vi "Turbulence_3.2.vi"() -> ()   [LabVIEW 2018]
uses:
  <instrlib>/Mercury iXX/Public/Controls/Comms Transport Layer.ctl
  <userlib>/LightField Add-in and Automation SDK/Samples/LabVIEW Automation/lightfield-automation-labview/LightField Automation.lvclass
  C:/Program Files/Princeton Instruments/LightField/AddInViews/PrincetonInstruments.LightFieldViewV3.dll
  Program Files/Princeton Instruments/LightField/AddInViews/PrincetonInstruments.LightFieldViewV3.dll
  C:/Program Files/Princeton Instruments/LightField/PrincetonInstruments.LightFieldAddInSupportServices.dll
  Program Files/Princeton Instruments/LightField/PrincetonInstruments.LightFieldAddInSupportServices.dll
  <instrlib>/Keithley 2600 Series/Public/Channel.ctl
  <vilib>/DAQmx/read.llb/DAQmx Read (Counter DBL 1Chan 1Samp).vi
  <instrlib>/Mercury iXX/Public/Libraries/System/Open/Open System.vi
  <instrlib>/Mercury iXX/Public/Libraries/System/Read/Catalogue (Read).vi
  <vilib>/DAQmx/miscellaneous.llb/DAQmx Fill In Error Info.vi
  <instrlib>/Mercury iXX/Public/Libraries/Temperature/Open/Open Temperature Device.vi
  <instrlib>/Mercury iXX/Public/Libraries/Temperature/Signals/Read/Temperature (Read).vi
  <instrlib>/Quantum Composers 9000 Series 2.08/Quantum Composers 9000 Series.lvlib
  <instrlib>/Mercury iXX/Mercury iXX.lvlib
  <instrlib>/Mercury iXX/Public/Libraries/Temperature.lvlib
  <instrlib>/Keithley 2600 Series/Keithley 2600 Series.lvlib
  <instrlib>/Mercury iXX/Public/Libraries/System.lvlib
panel:
  out "Low Level\n(Ohms)":dbl format="%.1f"
  out "High Level\n(Ohms)":dbl format="%.1f"
  in  "Second Gate Width (us)":dbl=0.3
  in  "Initial Gate Width (us)":dbl=0.3
  in  "Second Gate Delay (us)":dbl=999.7
  in  "Initial Gate Delay (us)":dbl=1001.4
  in  "Extra Waits":i32
  in  "Error":bool
  in  "3He Check":bool=TRUE
  in  "File Exists":bool=TRUE
  out "Log":refnum<file>
  in  "Motor free":bool
  in  "RESTART":bool
  out "time string":string="12:58:38 PM"
  out "Timestamp":string
  out "Log Error":errorcluster
  in  "CLOSE":bool
  in  "RECORD":bool
  in  "Turbulence":T1(tab)
  out "Translation Error":bool caption="Error"
  in  "Camera Set":dbl=15.0 min=0.0 max=18.5 step=0.01 format="%.2f"
  in  "Mirror Set":dbl=10.0 min=0.0 max=25.4 step=0.01 format="%.2f"
  out "Camera":dbl=15.0 format="%.2f"
  out "Mirror":dbl=10.0 format="%.2f"
  in  "Home":bool
  in  "FROM FILE":bool
  in  "Script File":path
  in  "# Frames":i32=1000 min=0 step=1
  in  "New Background Movie":bool
  in  "On CCD Acc.":i32=3 min=0 step=1
  in  "Cycle time\n(ms)":i32=15 min=0 step=1
  in  "New Background Frame":bool
  out "Rate (Hz)":dbl
  out "Incident":dbl
  in  "BIN":u16(ring)=2 items=["1x1", "2x2", "4x4"]
  in  "MODE":u16(ring)=1 items=["Normal", "DIF"]
  in  "Enable":bool
  out "Rate (Hz)":dbl
  out "Detected":dbl
  in  "Script\nEnd":u32=1 step=1
  in  "Sample Space Pump":bool
  in  "Siphon Pump":bool
  in  "Neutron Shutter":bool
  in  "Manual Script Entry (0)":string
  in  "READY":bool=TRUE
  out "Power (mW)":dbl format="%_3f"
  out "Tank P2 (Torr)":string="0"
  in  "LIGHTFIELD":bool
  in  "SCRIPTING":bool
  in  "Top Coil":bool
  out "Tank P1 (Torr)":string="0.0"
  out "Cell (K)":dbl format="%.3f"
  out "Cryostat (K)":dbl format="%.3f"
  in  "Data Interval (s)":dbl=0.5 min=0.4 max=10.0 step=0.05
  in  "RUN/STOP":bool
  in  "Bottom Coil":bool
  in  "Bottom Coil (mA)":dbl min=-1000.0 max=1000.0 step=1e-05
  in  "Top Coil (mA)":dbl min=-1000.0 max=1000.0 step=1e-05
  in  "Percent Open":i32 min=0 max=100 step=5
  in  "COOLDOWN":bool
  in  "Script\n#":i32 step=1
  in  "Kill Switch":bool
  in  "DATA":bool
  out "Scripting Error":T2
  in  "Shutter Mode":u16(ring)=1 items=["Manual"=1, "XGate"=5]
  in  "REFILL":bool
  in  "AUTOFILL":bool
  in  "Low Level":dbl=10.0 format="%#_13g"
  out "L-He Level":dbl(slide) scale=0.0..100.0
  out "Liquid Level":dbl format="%_2f"
  out "Homing":bool
  in  "High Level":dbl=10.0 format="%#_13g"
  in  "Top":bool caption="Top Level"
  in  "Middle":bool
  in  "Bottom":bool
  in  "Fill":bool
  in  "Tare":bool
  out "Actual 3He\nTank Pressure":dbl min=0.0 max=100.0 step=5.0 format="%#.1g"
  out "Desired V2\nPressure (3He)":dbl min=0.0 max=100.0 step=5.0 format="%#.1f"
  in  "Desired Tank\nPressure (3He)":dbl min=0.0 max=100.0 step=0.01 format="%#.2f"
  in  "Log Pressure":bool
  out "4He Pressure (Torr)":string="-0.1"
  out "3He Pressure (Torr)":string="1"
  in  "Fill Time (s)":u32=10
  out "Overall Error":T3={"status"=TRUE, "codes"=-1073807343, "source"="VISA Open in Mercury iXX.lvlib:System.lvlib:Open System.vi->Turbulence_3.2.vi"}
  # "Camera Controls"
  # "Temperature Readout"
  # "Translation Controls"
  # "Neutron Counts"
  # "Automation"
  # "Pressure Readout"
  # "Relay Controls"
  # "Needle Valve Control"
  # "Heater Controls"
  # "Neutron Shutter"
  # "Optical Shutter"
  # "Siphon Pump"
  # "Laser Power Meter"
  # "Sample Space\nPump"
  # "V1 = 4075 mL"
  # "V2 = 15.5 mL"
  # "V3 = 78.8 mL"
  # "Quartz\nCell"
  # "4"
  # "3psi relief"
  # "MFC"
  # "V1"
  # "4L Tank"
  # "Turbo Pump"
  # "V2"
  # "V3"
  # "3"
  # "10psi relief"
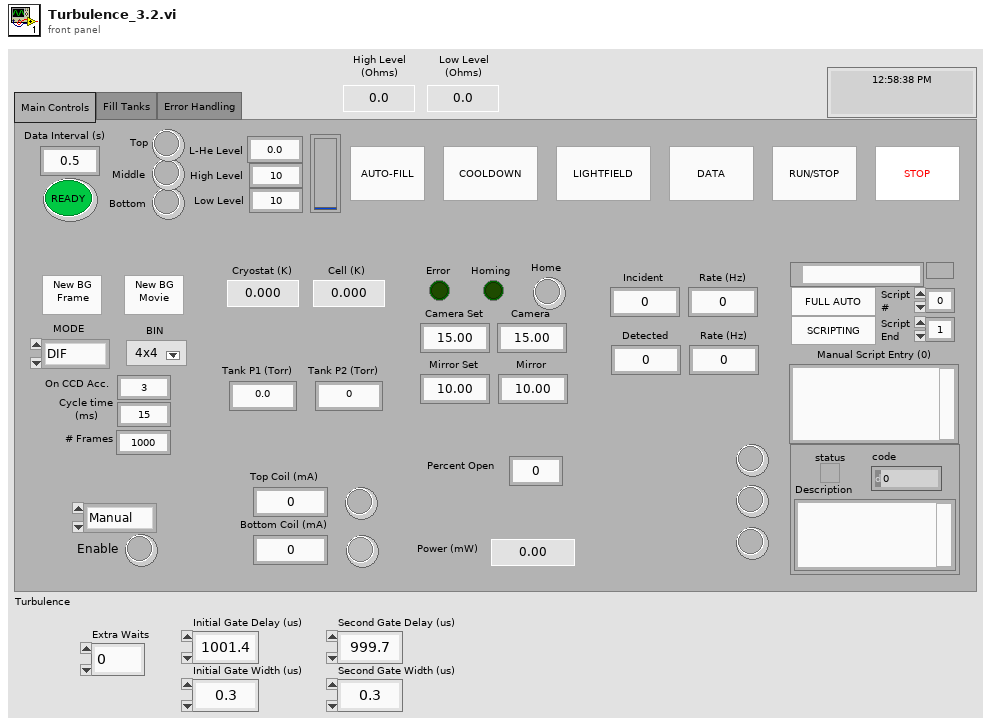
[diagram p1: front panel]
types:
  T1 = enum32{"Main Controls", "Fill Tanks", "Error Handling"}
  T2 = cluster{"status":bool, "code":i32, "Description":string}
  T3 = cluster{"status":bool, "codes":i32, "source":string}
  T4 = typedef "Mercury iXX.lvlib/Comms Transport Layer.ctl" = enum16{"Ethernet TCP/IP", "USB", "ISOBus - RS-232", "GPIB"}
  T5 = typedef "Mercury iXX.lvlib/Mercury Reference.ctl" = cluster{"Comms":refnum<visa-resource-name>, "Device ID":string[], "Comms Layer":T4, "Command":string, "Query reference":T6}
  T6 = typedef "Mercury iXX.lvlib/Query Dynamic Reference.ctl" = refnum<vi>
  T7 = enum32{"Current", "Voltage", "IV", "Resistance", "Power"}
  T8 = typedef "Keithley 2600 Series.lvlib/Channel.ctl" = enum32{"Channel A", "Channel B"}
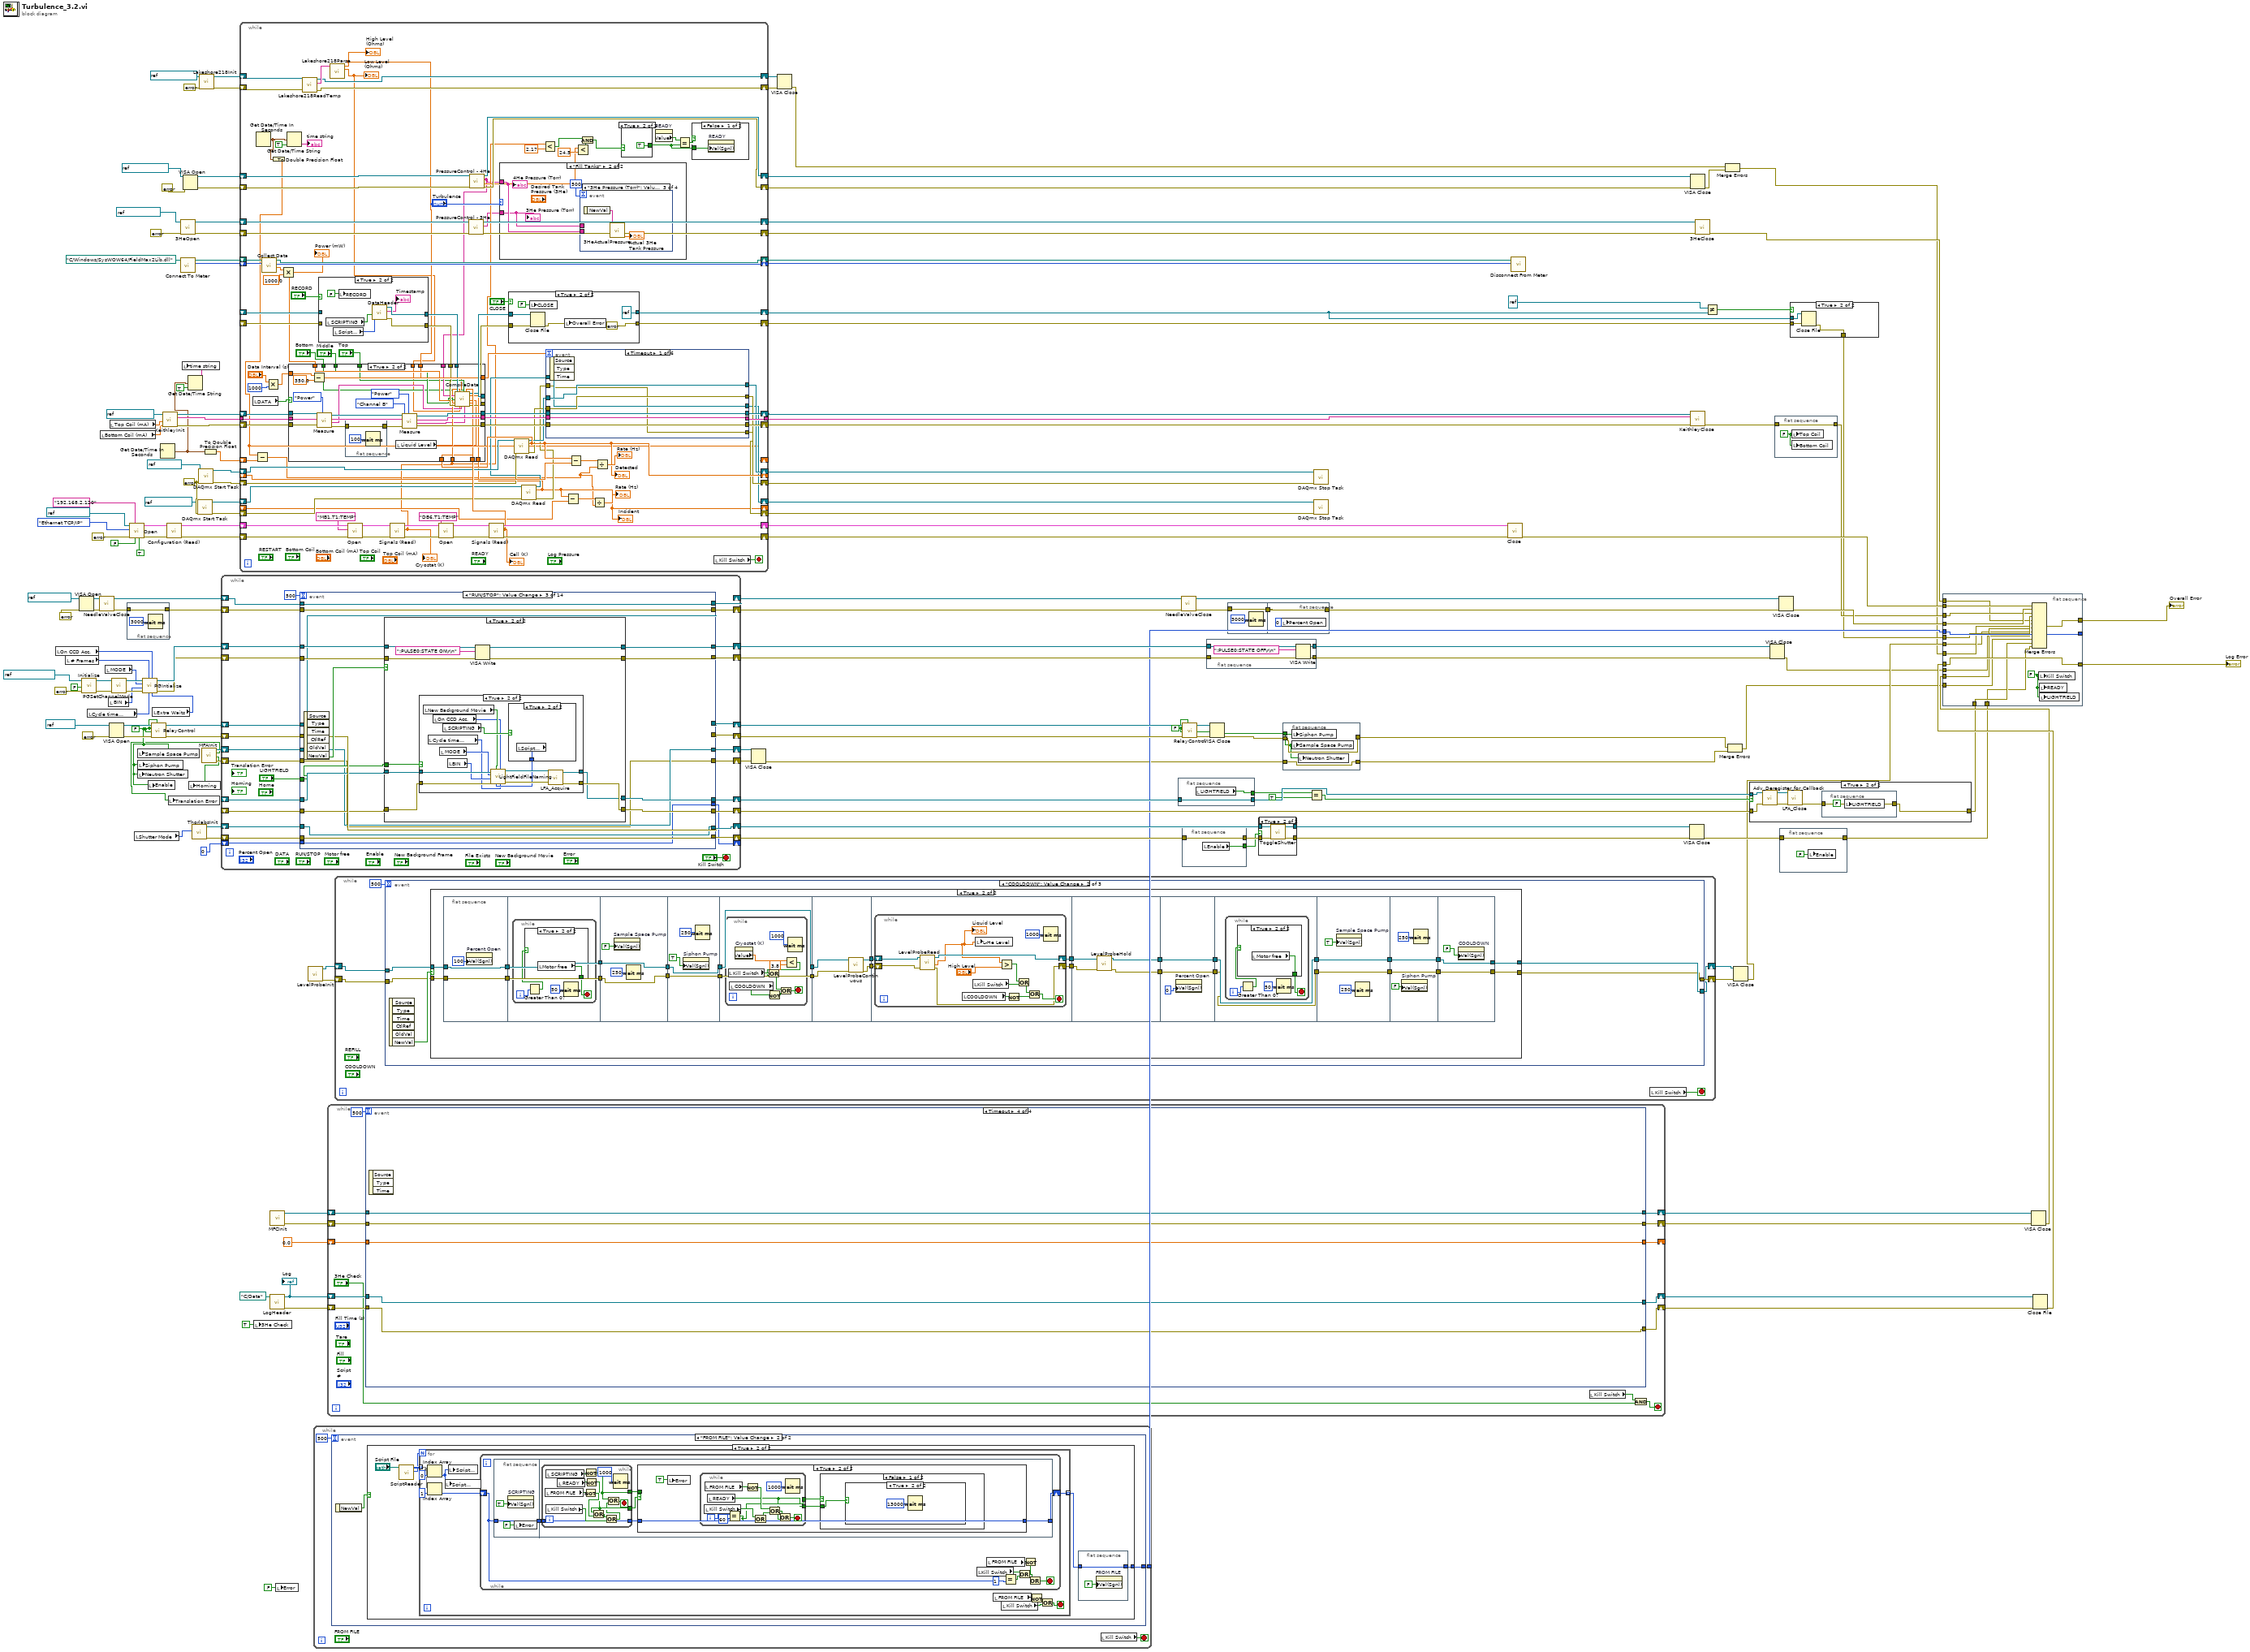
[diagram p0: block diagram]
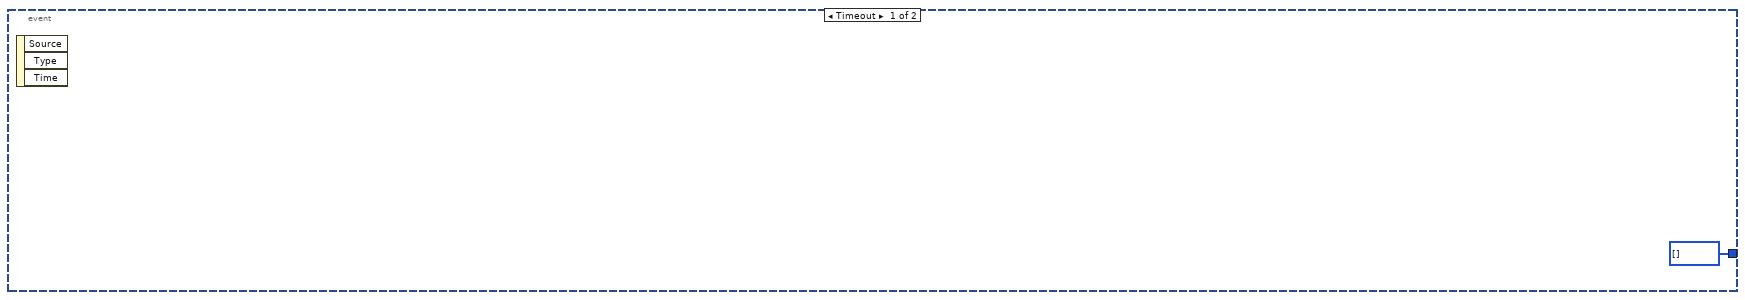
[diagram p2: hidden frame]
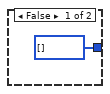
[diagram p3: hidden frame]
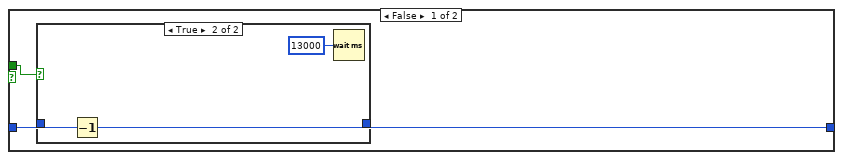
[diagram p4: hidden frame]
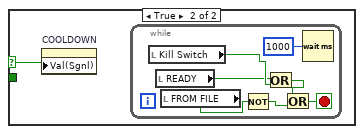
[diagram p7: hidden frame]
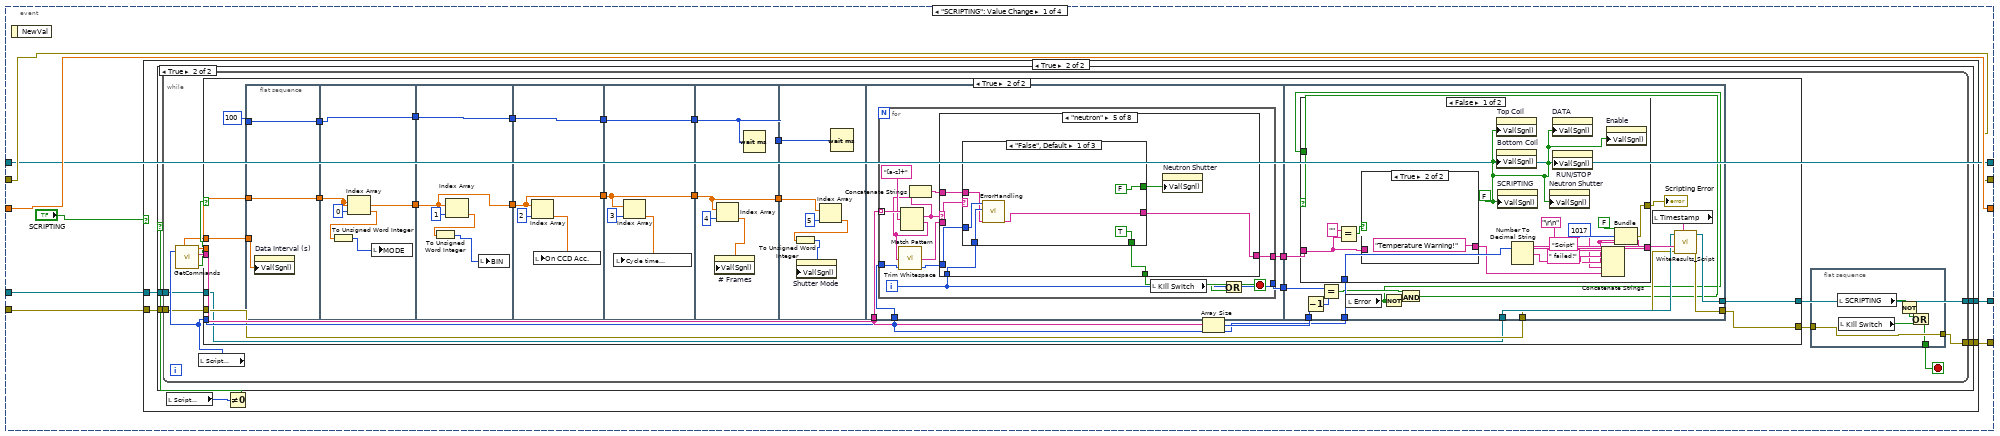
[diagram p10: hidden frame]
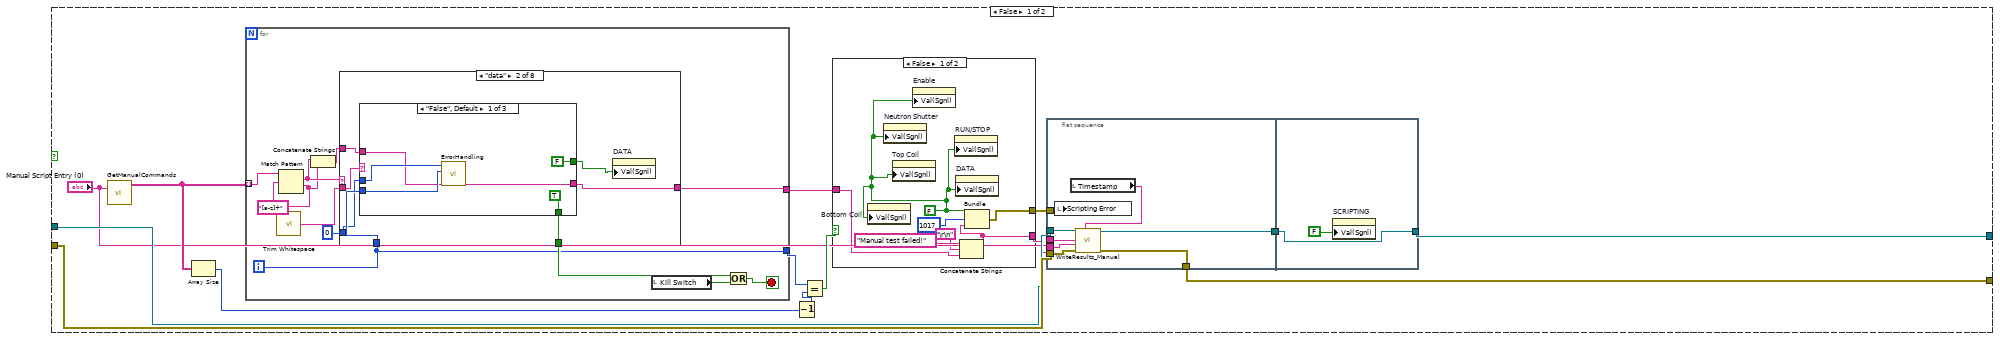
[diagram p12: hidden frame]
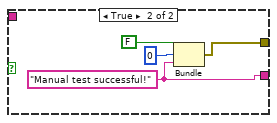
[diagram p13: hidden frame]
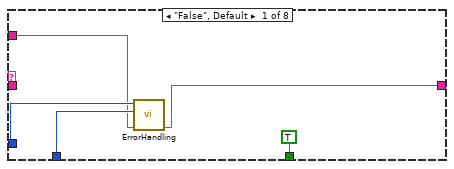
[diagram p14: hidden frame]
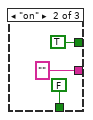
[diagram p15: hidden frame]
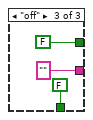
[diagram p16: hidden frame]
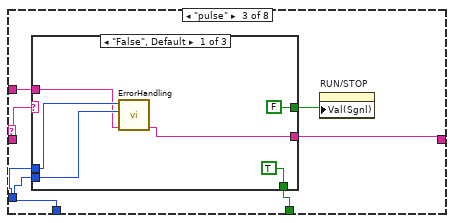
[diagram p17: hidden frame]
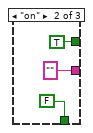
[diagram p18: hidden frame]
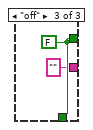
[diagram p19: hidden frame]
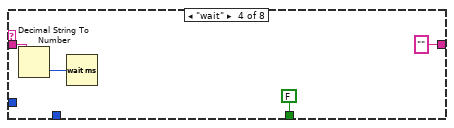
[diagram p20: hidden frame]
diagram:
  w65 = errorcluster {"status"=FALSE, "code"=0, "source"=""} ("error in")
  w101 = FALSE ("Siphon Pump")
  w87 = FALSE ("Siphon Pump")
  n1 = local read "On CCD Acc."() -> (w76:i32)
  n2 = local read "# Frames"() -> (w75:i32)
  n3 = VISA Open(error in (no error)=errorcluster {"status"=FALSE, "code"=0, "source"=""}, VISA resource name=refnum<visa-resource-name> "ZaberMotor") -> (VISA resource name=w82:refnum<visa-resource-name>, error out=w83:errorcluster)  [unwired: 3 in]
  n4 = call <instrlib>:"Initialize.vi"("error in (no error)"=errorcluster {"status"=FALSE, "code"=0, "source"=""}, "Reset? (T: Yes)"=FALSE, "VISA resource name"=refnum<visa-resource-name> "PulseGenerator" ("Pulse generater (COM3)")) -> ("error out"=w94:errorcluster, "VISA resource name out"=w92:refnum<visa-resource-name>)  [unwired: 7 in]
  n5 = local read "Cycle time\n(ms)"() -> (w44:i32)
  n6 = call "NeedleValveClose.vi"("error in (no error)"=w83, "VISA resource name"=w82) -> ("error out"=w84:errorcluster, "VISA resource name out"=w122:refnum<visa-resource-name>)  [unwired: 8 in]
  n7 = local read "Bottom Coil (mA)"() -> (w131:dbl)
  n8 = local read "MODE"() -> (w73:u16)
  n9 = local read "BIN"() -> (w74:u16)
  n10 = VISA Open(error in (no error)=errorcluster {"status"=FALSE, "code"=0, "source"=""} ("error in (no error) 2"), VISA resource name=refnum<visa-resource-name> "Relays" ("Pressure Gauge")) -> (VISA resource name=w143:refnum<visa-resource-name>, error out=w145:errorcluster)  [unwired: 3 in]
  n11 = local read "Top Coil (mA)"() -> (w132:dbl)
  n12 = call "PGSetChannelMode.vi"("error in"=w94, "VISA resource name"=w92) -> ("error out"=w93:errorcluster, "VISA resource name out"=w91:refnum<visa-resource-name>)  [unwired: 8 in]
  n13 = flat-sequence {
    tunnel: w84 -> [w170]
    tunnel: [w170] -> w123
    frame #0 {
      n14 = Wait (ms)(milliseconds to wait=u32 3000) -> ()  [unwired: 1 out]
    }
  }
  n15 = call-poly <instrlib>:"Open.vi"("Clear Previous Connections (False)"=TRUE, "ID Query (True)"=FALSE, "IP Address"="192.168.2.120", "error in (no error)"=errorcluster {"status"=FALSE, "code"=0, "source"=""}, "Comms Layer"=Comms_Transport_Layer."Ethernet TCP/IP", "VISA resource name"=refnum<visa-resource-name> "MercuryiTC") -> ("error out"=w163:errorcluster, "Mercury Reference Out"=w164:T5)  [unwired: 1 in, 3 out]
  n16 = local read "Shutter Mode"() -> (w77:u16)
  n17 = local write "Sample Space Pump"(w87) -> ()
  n18 = local write "Neutron Shutter"(w87) -> ()
  n19 = local write "Siphon Pump"(w87) -> ()
  n20 = local write "Enable"(w87) -> ()
  n21 = call "RelayControl.vi"("Neutron Shutter"=w87, "Error In"=w145, "Sample Space Pump"=w87, "Siphon Pump"=w87, "Relay In"=w143) -> ("Error Out"=w144:errorcluster, "Relay Out"=w142:refnum<visa-resource-name>)  [unwired: 5 in]
  n22 = local read "Extra Waits"() -> (w33:i32)
  n23 = call "PGIntialize.vi"("Extra Waits"=w33, "On CCD Accumulations"=w76, "Cycle time\n(ms)"=w44, "Number of Frames"=w75, "error in"=w93, "BIN"=w74, "MODE"=w73, "VISA resource name"=w91) -> ("error out"=w167:errorcluster, "VISA resource name out"=w168:refnum<visa-resource-name>)  [unwired: 2 in]
  n24 = Get Date/Time In Seconds() -> (seconds since 1Jan1904=w45:timestamp)
  n25 = call "KeithleyInit.vi"("Bottom Coil (mA)"=w131, "Top Coil (mA)"=w132, "KeithleyVISA In"=refnum<visa-resource-name> "Keithley2614B" ("VISA resource name")) -> ("error out"=w135:errorcluster, "Node Out"=w136:string, "KeithleyVISA Out"=w134:refnum<visa-resource-name>)  [unwired: 6 in]
  n26 = call-poly <instrlib>:"Configuration (Read).vi"("error in"=w163, "Mercury Reference In"=w164) -> ("error out"=w159:errorcluster, "Mercury Reference Out"=w160:T5)  [unwired: 6 in, 2 out]
  n27 = call "Connect To Meter.vi"("Location of FieldMax2Lib.dll in"=path "C:/Windows/SysWOW64/FieldMax2Lib.dll") -> ("Meter ID out"=w109:i32, "Location of FieldMax2Lib.dll out"=w108:path)  [unwired: 6 in, 1 out]
  n28 = call "3HeOpen.vi"("error in (no error)"=errorcluster {"status"=FALSE, "code"=0, "source"=""} ("error in (no error) 2"), "VISA resource name"=refnum<visa-resource-name> "3HePressure" ("Pressure Gauge")) -> ("error out"=w147:errorcluster, "VISA resource name out"=w146:refnum<visa-resource-name>)  [unwired: 8 in]
  n29 = VISA Open(error in (no error)=errorcluster {"status"=FALSE, "code"=0, "source"=""} ("error in (no error) 2"), VISA resource name=refnum<visa-resource-name> "TankPressure" ("Pressure Gauge")) -> (VISA resource name=w156:refnum<visa-resource-name>, error out=w157:errorcluster)  [unwired: 3 in]
  n30 = Get Date/Time String(seconds (now)=w45, want seconds? (F)=TRUE) -> (time string=w46:string)  [unwired: 1 in, 1 out]
  n31 = local write "time string"(w46) -> ()
  n32 = call "ThorlabsInit.vi"("Shutter Mode"=w77) -> ("error out"=w88:errorcluster, "VISA resource name out"=w89:refnum<visa-resource-name>)  [unwired: 9 in]
  n33 = call <vilib>:"DAQmx Start Task.vi"("task/channels in"=refnum<k21> "IncidentBeam", "error in"=w65) -> ("task out"=w67:refnum<k21>, "error out"=w66:errorcluster)  [unwired: 12 in]
  n34 = call <vilib>:"DAQmx Start Task.vi"("task/channels in"=refnum<k21> "Detector", "error in"=w65) -> ("task out"=w70:refnum<k21>, "error out"=w69:errorcluster)  [unwired: 12 in]
  n35 = call "Lakeshore218Init.vi"("error in (no error)"=errorcluster {"status"=FALSE, "code"=0, "source"=""}, "VISA resource name"=refnum<visa-resource-name> "Lakeshore218") -> ("error out"=w14:errorcluster, "VISA resource name out"=w15:refnum<visa-resource-name>)  [unwired: 8 in]
  n36 = call "MFAInit.vi"() -> ("error out"=w31:errorcluster, "Homing"=w25:bool, "Timeout"=w24:bool, "reference out"=w32:refnum<visa-resource-name>)  [unwired: 8 in]
  n37 = local write "Translation Error"(w24) -> ()
  n38 = local write "Homing"(w25) -> ()
  n39 = To Double Precision Float(number=w45) -> (double precision float=w48:dbl)
  n40 = while {
    shift-right: [w199] -> w55
    shift-left: _ -> [w197]
    shift-right: [w200] -> w61
    shift-left: _ -> [w198]
    shift-right: [w193] -> w116
    shift-left: w168 -> [w195]
    shift-right: [w194] -> w117
    shift-left: w167 -> [w196]
    shift-right: [w189] -> w121
    shift-left: w144 -> [w192]
    shift-right: [w190] -> w119
    shift-left: w142 -> [w191]
    shift-right: [w184] -> w148
    shift-left: w123 -> [w187]
    shift-right: [w185] -> w149
    shift-left: w122 -> [w186]
    shift-right: [w181] -> w57
    shift-left: w89 -> [w178]
    shift-right: [w180] -> w51
    shift-left: w88 -> [w179]
    shift-right: [w175] -> w30
    shift-left: w32 -> [w177]
    shift-right: [w174] -> w29
    shift-left: w31 -> [w176]
    shift-right: [w172] -> _
    shift-left: 0 -> [w173]
    stop <- "Kill Switch" stop-if-true
    n41 = event shown="[2] \"RUN/STOP\": Value Change" {
      selector: _ -> [_ _ _ _ _ _ _ _ _ _ _ _ _ _]
      dyn-events: _ -> [_ _ _ _ _ _ _ _ _ _ _ _ _ _]
      timeout: 500 -> [_ _ _ _ _ _ _ _ _ _ _ _ _ _]
      tunnel: w196 -> [w227 w252 w336 w385 w406 w458 w526 w548 w566 w592 w620 w677 w700 w735]
      tunnel: w195 -> [w226 w251 w337 w386 w405 w459 w527 w547 w565 w591 w621 w678 w701 w736]
      tunnel: w198 -> [w228 w255 w327 w377 w408 w462 w524 w551 w570 w583 w616 w673 w691 w733]
      tunnel: w197 -> [w229 w256 w328 w378 w409 w463 w525 w552 w569 w584 w617 w674 w692 w734]
      tunnel: [w228 w257 w326 w377 w408 w450 w524 w551 w570 w583 w616 w673 w691 w726] -> w200
      tunnel: [w229 w258 w325 w378 w409 w442 w525 w552 w569 w584 w617 w674 w692 w725] -> w199
      tunnel: [w227 w252 w339 w385 w406 w448 w526 w548 w566 w589 w620 w677 w700 w735] -> w194
      tunnel: [w226 w251 w338 w386 w405 w455 w527 w547 w565 w590 w621 w678 w701 w736] -> w193
      tunnel: w192 -> [w224 w253 w333 w383 w411 w457 w533 w550 w568 w585 w618 w675 w698 w728]
      tunnel: w191 -> [w225 w254 w334 w384 w410 w456 w532 w549 w567 w586 w619 w676 w699 w727]
      tunnel: [w225 w254 w334 w384 w410 w456 w529 w549 w567 w586 w619 w676 w699 w727] -> w190
      tunnel: [w224 w253 w333 w383 w411 w457 w528 w550 w568 w585 w618 w675 w698 w728] -> w189
      tunnel: w187 -> [w223 w250 w332 w387 w394 w461 w523 w546 w564 w587 w622 w679 w702 w737]
      tunnel: w186 -> [w222 w249 w331 w388 w407 w460 w522 w545 w563 w588 w623 w680 w703 w738]
      tunnel: [w222 w249 w331 w388 w404 w460 w522 w545 w563 w588 w623 w680 w703 w738] -> w185
      tunnel: [w223 w250 w332 w387 w396 w461 w523 w546 w564 w587 w622 w679 w702 w737] -> w184
      tunnel: "LIGHTFIELD" -> [_ _ w324 w382 _ w444 _ _ _ w579 _ _ _ w724]
      tunnel: w178 -> [w220 w247 w330 w380 w402 w454 w520 w544 w574 w582 w615 w672 w690 w732]
      tunnel: w179 -> [w221 w246 w329 w379 w401 w453 w519 w543 w573 w581 w614 w671 w689 w731]
      tunnel: [w220 w247 w330 w380 w402 w454 w520 w541 w571 w582 w615 w672 w690 w732] -> w181
      tunnel: [w221 w246 w329 w379 w401 w453 w519 w542 w572 w581 w614 w671 w689 w731] -> w180
      tunnel: w177 -> [w210 w245 w323 w376 w393 w439 w516 w537 w561 w577 w613 w667 w694 w729]
      tunnel: w176 -> [w211 w244 w322 w375 w392 w438 w515 w536 w560 w576 w612 w666 w693 w730]
      tunnel: [w212 w245 w323 w376 w393 w439 w516 w537 w561 w577 w613 w665 w688 w729] -> w175
      tunnel: [w207 w244 w322 w375 w392 w438 w515 w536 w560 w576 w612 w664 w687 w730] -> w174
      tunnel: w173 -> [w202 w243 w321 w374 w391 w437 w514 w535 w559 w575 w611 w659 w685 w723]
      tunnel: [w201 w243 w321 w374 w391 w437 w514 w535 w559 w575 w611 w659 w685 w723] -> w172
      event Timeout {
        n42 = event-data() -> ()  [unwired: 1 in, 3 out]
        n43 = call <instrlib>:"tell current position.vi"("error in"=w211, "Axis in"=1, "VISA Handle in"=w210) -> ("error out"=w208:errorcluster, "Current position (units)"=w204:dbl, "VISA Handle out"=w218:refnum<visa-resource-name>, "TimeoutFlag"=w216:bool)  [unwired: 2 in, 1 out]
        "Camera" <- w204
        n44 = flat-sequence {
          tunnel: w208 -> [w242]
          tunnel: [w242] -> w213
          frame #0 {
            n45 = Wait (ms)(milliseconds to wait=u32 50) -> ()  [unwired: 1 out]
          }
        }
        n46 = call <instrlib>:"tell current position.vi"("error in"=w213, "Axis in"=2, "VISA Handle in"=w218) -> ("error out"=w207:errorcluster, "Current position (units)"=w203:dbl, "VISA Handle out"=w212:refnum<visa-resource-name>, "TimeoutFlag"=w215:bool)  [unwired: 2 in, 1 out]
        "Mirror" <- w203
        n47 = Or(x=w216, y=w215) -> (x .or. y?=w214:bool)
        n48 = local write "Translation Error"(w214) -> ()
        n49 = local read "Homing"() -> (w209:bool)
        n50 = Equal?(x=w202, y=0) -> (x = y?=w206:bool)
        n51 = case shown="True" w209 {
          tunnel: w203 -> [_ w235]
          tunnel: w204 -> [_ w234]
          frame False {
          }
          frame True {
            w236 = 0.0 ("y")
            n52 = Equal?(x=w235, y=w236) -> (x = y?=w239:bool)
            n53 = Equal?(x=w234, y=w236) -> (x = y?=w238:bool)
            n54 = And(x=w239, y=w238) -> (x .and. y?=w237:bool)
            n55 = case shown="False" w237 {
              frame False {
              }
              frame True {
                n56 = local write "Homing"(FALSE ("Homing")) -> ()
              }
            }
          }
        }
        n57 = case shown="True" w206 {
          tunnel: w204 -> [_ w232]
          tunnel: w203 -> [_ w231]
          tunnel: w202 -> [w230 _]
          tunnel: [w230 1] -> w201
          frame False {
          }
          frame True {
            n58 = local write "Camera Set"(w232) -> ()
            n59 = local write "Mirror Set"(w231) -> ()
          }
        }
      }
      event "LIGHTFIELD": Value Change {
        n60 = event-data() -> ("NewVal"=w248:bool)  [unwired: 1 in, 5 out]
        n61 = case shown="False" w248 {
          tunnel: [refnum<class "LightField Automation.lvclass"> refnum ("LightField Automation out") w274] -> w258
          tunnel: [errorcluster {"status"=FALSE, "code"=0, "source"=""} ("error out") w273] -> w257
          tunnel: w256 -> [w263 _]
          tunnel: w255 -> [w262 _]
          frame False {
            n62 = call <userlib>:"Adv_Deregister_for_Callback.vi"("error in (no error)"=w262, "LightField Automation in"=w263) -> ("error out"=w264:errorcluster, "LightField Automation out"=w265:refnum<class "LightField Automation.lvclass">)  [unwired: 8 in]
            n63 = call <userlib>:"LFA_Close.vi"("error in (no error)"=w264, "LightField Automation in"=w265) -> ("error out"=w259:errorcluster)  [unwired: 8 in, 1 out]
            n64 = local write "Overall Error"(w259) -> ()
          }
          frame True {
            n65 = call <userlib>:"LFA_Initialize.vi"("error in (no error)"=errorcluster {"status"=FALSE, "code"=0, "source"=""}) -> ("error out"=w283:errorcluster, "LightField Automation out"=w282:refnum<class "LightField Automation.lvclass">)  [unwired: 9 in]
            n66 = call <userlib>:"Adv_Register_for_Callback.vi"("error in (no error)"=w283, "LightField Automation in"=w282) -> ("error out"=w281:errorcluster, "LightField Automation out"=w280:refnum<class "LightField Automation.lvclass">)  [unwired: 8 in]
            n67 = call <userlib>:"Exp_SetExperiment.vi"("error in (no error)"=w281, "ExperimentName"="20190801_DIF", "LightField Automation in"=w280) -> ("error out"=w267:errorcluster, "LightField Automation out"=w266:refnum<class "LightField Automation.lvclass">)  [unwired: 7 in]
            n68 = flat-sequence {
              tunnel: [w291] -> w271
              tunnel: [w290] -> w270
              tunnel: [w289] -> w269
              tunnel: [w292] -> w268
              tunnel: w267 -> [w295]
              tunnel: w266 -> [w293]
              tunnel: [w306] -> w277
              tunnel: [w305] -> w276
              tunnel: [w304] -> w275
              tunnel: [w303] -> w272
              tunnel: w271 -> [w303]
              tunnel: w270 -> [w306]
              tunnel: w269 -> [w305]
              tunnel: w268 -> [w304]
              tunnel: w277 -> [w311]
              tunnel: w276 -> [w312]
              tunnel: w275 -> [w310]
              tunnel: [w309] -> w274
              tunnel: [w308] -> w273
              tunnel: w272 -> [w307]
              frame #0 {
                n69 = local read "On CCD Acc."() -> (w301:i32)
                n70 = local read "Cycle time\n(ms)"() -> (w288:i32)
                n71 = local read "# Frames"() -> (w299:i32)
                n72 = local read "Second Gate Width (us)"() -> (w285:dbl)
                n73 = local read "BIN"() -> (w300:u16)
                n74 = local read "Second Gate Delay (us)"() -> (w284:dbl)
                n75 = local read "Initial Gate Width (us)"() -> (w286:dbl)
                n76 = call <userlib>:"Exp_ICCD_SetIntensifierGain.vi"("error in (no error)"=w295, "Intensifier Gain"=100, "LightField Automation in"=w293) -> ("error out"=w297:errorcluster, "LightField Automation out"=w296:refnum<class "LightField Automation.lvclass">)  [unwired: 7 in]
                n77 = local read "Initial Gate Delay (us)"() -> (w287:dbl)
                n78 = local read "MODE"() -> (w302:u16)
                n79 = local read "Log"() -> (w298:refnum<file>)
                n80 = call "LightFieldInit.vi"("LightField Automation in"=w296, "MODE"=w302, "BIN"=w300, "error in"=w297, "Initial Gate Delay (us)"=w287, "Initial Gate Width (us)"=w286, "Number of Frames"=w299, "File Path"=w298, "On CCD Accumulations"=w301, "Second Gate Delay (us)"=w284, "Second Gate Width (us)"=w285) -> ("LightField Automation out"=w289:refnum<class "LightField Automation.lvclass">, "error out"=w290:errorcluster)  [unwired: 7 in]
                n81 = call "LightFieldBackgroundNaming.vi"("Cycle time\n(ms)"=w288, "On CCD Acc."=w301, "BIN"=w300, "MODE"=w302) -> ("FilePath"=w292:string, "Exists"=w291:bool)  [unwired: 5 in, 1 out]
              }
              frame #1 {
                n82 = local write "File Exists"(w303) -> ()
              }
              frame #2 {
                n83 = case shown="False" w307 {
                  tunnel: w312 -> [w315 w320]
                  tunnel: w311 -> [w314 w319]
                  tunnel: w310 -> [_ w318]
                  tunnel: [w315 w317] -> w309
                  tunnel: [w314 w316] -> w308
                  frame False {
                    n84 = property on="New Background Frame" class="Bool (strict)"("Val(Sgnl)"=TRUE ("Value (Signaling)")) -> ()  [unwired: 2 in, 2 out]
                  }
                  frame True {
                    n85 = call "LightFieldChangeBackground.vi"("error in"=w319, "FilePath"=w318, "LightField Automation in"=w320) -> ("error out"=w316:errorcluster, "LightField Automation out"=w317:refnum<class "LightField Automation.lvclass">)  [unwired: 7 in]
                  }
                }
              }
            }
          }
        }
      }
      event "RUN/STOP": Value Change {
        n86 = event-data() -> ("NewVal"=w335:bool)  [unwired: 1 in, 5 out]
        n87 = case shown="True" w335 {
          tunnel: [w343 w356] -> w339
          tunnel: [w344 w355] -> w338
          tunnel: w337 -> [w345 w354]
          tunnel: w336 -> [w346 w353]
          tunnel: w328 -> [w341 w351]
          tunnel: w327 -> [w340 w350]
          tunnel: [w340 w349] -> w326
          tunnel: [w341 w348] -> w325
          tunnel: w324 -> [_ w347]
          frame False {
            n88 = VISA Write(VISA resource name=w345, write buffer=":PULSE0:STATE OFF\r\n" ("format string"), error in (no error)=w346) -> (VISA resource name out=w344:refnum<visa-resource-name>, error out=w343:errorcluster)  [unwired: 1 out]
          }
          frame True {
            n89 = case shown="True" w347 {
              tunnel: w350 -> [w357 w369]
              tunnel: w351 -> [w358 w367]
              tunnel: [w358 w371] -> w348
              tunnel: [w357 w370] -> w349
              frame False {
              }
              frame True {
                n90 = local read "New Background Movie"() -> (w361:bool)
                n91 = local read "Cycle time\n(ms)"() -> (w359:i32)
                n92 = local read "On CCD Acc."() -> (w360:i32)
                n93 = local read "MODE"() -> (w364:u16)
                n94 = local read "SCRIPTING"() -> (w362:bool)
                n95 = local read "BIN"() -> (w365:u16)
                n96 = case shown="True" w362 {
                  tunnel: [-1 ("Script\n#") w373] -> w363
                  frame False {
                  }
                  frame True {
                    n97 = local read "Script\n#"() -> (w373:i32)
                  }
                }
                n98 = call "LightFieldFileNaming.vi"("Cycle time\n(ms)"=w359, "On CCD Acc."=w360, "Script#"=w363, "BG"=w361, "error in"=w369, "BIN"=w365, "MODE"=w364, "LightField Automation in"=w367) -> ("error out"=w368:errorcluster, "LightField Automation out"=w366:refnum<class "LightField Automation.lvclass">)  [unwired: 2 in]
                n99 = call <instrlib>:"LFA_Acquire.vi"("error in (no error)"=w368, "LightField Automation in"=w366) -> ("error out"=w370:errorcluster, "LightField Automation out"=w371:refnum<class "LightField Automation.lvclass">)  [unwired: 8 in]
              }
            }
            n100 = VISA Write(VISA resource name=w354, write buffer=":PULSE0:STATE ON\r\n" ("format string"), error in (no error)=w353) -> (VISA resource name out=w355:refnum<visa-resource-name>, error out=w356:errorcluster)  [unwired: 1 out]
          }
        }
      }
      event "DATA": Value Change {
        n101 = event-data() -> ("NewVal"=w381:bool)  [unwired: 1 in, 5 out]
        n102 = case shown="False" w381 {
          tunnel: w382 -> [_ _]
          frame False {
            n103 = local write "CLOSE"(TRUE ("CLOSE")) -> ()
          }
          frame True {
            n104 = local write "RECORD"(TRUE ("RECORD")) -> ()
          }
        }
      }
      event "Percent Open": Value Change {
        n105 = event-data() -> ("OldVal"=w403:i32, "NewVal"=w412:i32)  [unwired: 1 in, 4 out]
        n106 = flat-sequence {
          tunnel: w394 -> [w414]
          tunnel: [w414] -> w395
          frame #0 {
            n107 = property on="Motor free" class="Bool (strict)"("Val(Sgnl)"=FALSE ("Value (Signaling)")) -> ()  [unwired: 2 in, 2 out]
          }
        }
        n108 = Subtract(x=w412, y=w403) -> (x-y=w398:i32)
        n109 = Greater Than 0?(x=w398) -> (x > 0?=w399:bool)
        n110 = Equal To 0?(x=w412) -> (x = 0?=w400:bool)
        n111 = case shown="False" w400 {
          tunnel: w407 -> [w420 w436]
          tunnel: w395 -> [w421 w435]
          tunnel: [w419 w434] -> w404
          tunnel: [w418 w433] -> w397
          tunnel: w399 -> [w422 _]
          tunnel: w398 -> [w417 _]
          frame False {
            n112 = case shown="True" w422 {
              tunnel: w421 -> [w426 w432]
              tunnel: w420 -> [w427 w431]
              tunnel: [w425 w430] -> w419
              tunnel: [w424 w429] -> w418
              tunnel: w417 -> [w423 w428]
              frame False {
                n113 = call "NeedleValveClose - Encoder.vi"("error in (no error)"=w426, "Percent Difference"=w423, "VISA resource name"=w427) -> ("error out"=w424:errorcluster, "VISA resource name out"=w425:refnum<visa-resource-name>)  [unwired: 7 in]
              }
              frame True {
                n114 = call "NeedleValveOpen - Encoder.vi"("error in (no error)"=w432, "Percent Difference"=w428, "VISA resource name"=w431) -> ("error out"=w429:errorcluster, "VISA resource name out"=w430:refnum<visa-resource-name>)  [unwired: 7 in]
              }
            }
          }
          frame True {
            n115 = call "NeedleValveClose.vi"("error in (no error)"=w435, "VISA resource name"=w436) -> ("error out"=w433:errorcluster, "VISA resource name out"=w434:refnum<visa-resource-name>)  [unwired: 8 in]
          }
        }
        n116 = flat-sequence {
          tunnel: w397 -> [w416]
          tunnel: [w416] -> w396
          frame #0 {
            n117 = property on="Motor free" class="Bool (strict)"("Val(Sgnl)"=TRUE ("Value (Signaling)")) -> ()  [unwired: 2 in, 2 out]
          }
        }
      }
      event "Cycle time\n(ms)", "# Frames", "MODE", "BIN", "On CCD Acc.", "Extra Waits": Value Change {
        n118 = event-data() -> ()  [unwired: 1 in, 1 out]
        n119 = case shown="True" w444 {
          tunnel: w463 -> [w504 w512]
          tunnel: w462 -> [w505 w513]
          tunnel: [w504 w511] -> w443
          tunnel: [w505 w510] -> w451
          tunnel: "On CCD Acc." -> [_ w508]
          tunnel: "# Frames" -> [_ w509]
          tunnel: "BIN" -> [_ w507]
          tunnel: "MODE" -> [_ w506]
          frame False {
          }
          frame True {
            n120 = call "LightFieldParams.vi"("On CCD Accumulations"=w508, "Number of Frames"=w509, "error in"=w513, "BIN"=w507, "MODE"=w506, "LightField Automation in"=w512) -> ("error out"=w510:errorcluster, "LightField Automation out"=w511:refnum<class "LightField Automation.lvclass">)  [unwired: 4 in]
          }
        }
        n121 = call "PGIntialize.vi"("Extra Waits"="Extra Waits", "On CCD Accumulations"="On CCD Acc.", "Cycle time\n(ms)"="Cycle time\n(ms)", "Number of Frames"="# Frames", "error in"=w458, "BIN"="BIN", "MODE"="MODE", "VISA resource name"=w459) -> ("error out"=w449:errorcluster, "VISA resource name out"=w455:refnum<visa-resource-name>)  [unwired: 2 in]
        n122 = case shown="True" w444 {
          tunnel: w451 -> [w466 w476]
          tunnel: [w466 w475] -> w450
          tunnel: w449 -> [w465 w474]
          tunnel: [w465 w473] -> w448
          tunnel: "On CCD Acc." -> [_ w472]
          tunnel: "BIN" -> [_ w471]
          tunnel: "MODE" -> [_ w470]
          tunnel: w443 -> [w464 w469]
          tunnel: [w464 w468] -> w442
          tunnel: "Cycle time\n(ms)" -> [_ w467]
          frame False {
          }
          frame True {
            n123 = flat-sequence {
              tunnel: w476 -> [w480]
              tunnel: [w479] -> w475
              tunnel: w474 -> [w488]
              tunnel: [w488] -> w473
              tunnel: w472 -> [w487]
              tunnel: w471 -> [w486]
              tunnel: w470 -> [w485]
              tunnel: w469 -> [w481]
              tunnel: [w478] -> w468
              tunnel: w467 -> [w477]
              frame #0 {
                n124 = call "LightFieldBackgroundNaming.vi"("Cycle time\n(ms)"=w477, "On CCD Acc."=w487, "BIN"=w486, "MODE"=w485) -> ("FilePath"=w482:string, "Exists"=w484:bool)  [unwired: 5 in, 1 out]
                n125 = flat-sequence {
                  tunnel: w484 -> [w489]
                  tunnel: [w489] -> w483
                  tunnel: w483 -> [w495]
                  tunnel: w482 -> [w494]
                  tunnel: w481 -> [w493]
                  tunnel: w480 -> [w492]
                  tunnel: [w491] -> w479
                  tunnel: [w490] -> w478
                  frame #0 {
                    n126 = local write "File Exists"(w489) -> ()
                  }
                  frame #1 {
                    n127 = case shown="True" w495 {
                      tunnel: w494 -> [_ w503]
                      tunnel: w493 -> [w497 w502]
                      tunnel: w492 -> [w496 w501]
                      tunnel: [w496 w500] -> w491
                      tunnel: [w497 w499] -> w490
                      frame False {
                        n128 = property on="New Background Frame" class="Bool (strict)"("Val(Sgnl)"=TRUE ("Value (Signaling)")) -> ()  [unwired: 2 in, 2 out]
                      }
                      frame True {
                        n129 = call "LightFieldChangeBackground.vi"("error in"=w501, "FilePath"=w503, "LightField Automation in"=w502) -> ("error out"=w500:errorcluster, "LightField Automation out"=w499:refnum<class "LightField Automation.lvclass">)  [unwired: 7 in]
                      }
                    }
                  }
                }
              }
            }
          }
        }
      }
      event "Siphon Pump", "Sample Space Pump", "Neutron Shutter": Value Change {
        n130 = event-data() -> ("CtlRef"=w517:refnum<vi>)  [unwired: 1 in]
        n131 = property class="Bool (strict)"(reference=w517) -> ("Label.Text"=w518:string)  [unwired: 1 in, 2 out]
        n132 = call "RelayControl.vi"("Neutron Shutter"="Neutron Shutter", "Error In"=w533, "Sample Space Pump"="Sample Space Pump", "Siphon Pump"="Siphon Pump", "Relay In"=w532) -> ("Error Out"=w528:errorcluster, "Relay Out"=w529:refnum<visa-resource-name>)  [unwired: 5 in]
        n133 = case shown="\"Neutron Shutter\"" w518 {
          frame "0", Default {
          }
          frame "Neutron Shutter" {
            n134 = property on="RESTART" class="Bool (strict)"("Val(Sgnl)"=TRUE ("RESTART")) -> ()  [unwired: 2 in, 2 out]
          }
        }
      }
      event "Enable": Value Change {
        n135 = event-data() -> ("OldVal"=w539:bool, "NewVal"=w540:bool)  [unwired: 1 in, 4 out]
        n136 = Not Equal?(x=w539, y=w540) -> (x != y?=w538:bool)
        n137 = case shown="True" w538 {
          tunnel: w544 -> [w554 w558]
          tunnel: w543 -> [w553 w557]
          tunnel: [w553 w556] -> w542
          tunnel: [w554 w555] -> w541
          frame False {
          }
          frame True {
            n138 = call "ToggleShutter.vi"("error in"=w557, "VISA resource name"=w558) -> ("error out"=w556:errorcluster, "VISA resource name out"=w555:refnum<visa-resource-name>)  [unwired: 8 in]
          }
        }
      }
      event "Shutter Mode": Value Change {
        n139 = event-data() -> ()  [unwired: 1 in, 6 out]
        n140 = call "ThorlabsMode.vi"("error in"=w573, "Mode"="Shutter Mode", "VISA resource name"=w574) -> ("error out"=w572:errorcluster, "VISA resource name out"=w571:refnum<visa-resource-name>)  [unwired: 7 in]
      }
      event "New Background Frame": Value Change {
        n141 = event-data() -> ("NewVal"=w580:bool)  [unwired: 1 in]
        n142 = And(x=w580, y=w579) -> (x .and. y?=w578:bool)
        n143 = case shown="True" w578 {
          tunnel: w592 -> [w593 w606]
          tunnel: w591 -> [w594 w607]
          tunnel: [w594 w604] -> w590
          tunnel: [w593 w598] -> w589
          frame False {
          }
          frame True {
            n144 = local read "Cycle time\n(ms)"() -> (w596:i32)
            n145 = local read "On CCD Acc."() -> (w605:i32)
            n146 = local read "MODE"() -> (w601:u16)
            n147 = local read "File Exists"() -> (w597:bool)
            n148 = local read "Extra Waits"() -> (w595:i32)
            n149 = local read "BIN"() -> (w600:u16)
            n150 = call "LightFieldAcquireBackground.vi"("Cycle time\n(ms)"=w596, "File Exists"=w597, "On CCD Acc."=w605, "error in"=w606, "BIN"=w600, "MODE"=w601, "VISA resource name"=w607) -> ("error out"=w603:errorcluster, "VISA resource name out"=w602:refnum<visa-resource-name>)  [unwired: 3 in]
            n151 = call "PGResetCameraWait.vi"("Extra Waits"=w595, "Cycle time\n(ms)"=w596, "error in"=w603, "BIN"=w600, "MODE"=w601, "VISA resource name"=w602) -> ("error out"=w599:errorcluster, "VISA resource name out"=w604:refnum<visa-resource-name>)  [unwired: 4 in]
            n152 = flat-sequence {
              tunnel: w599 -> [w609]
              tunnel: [w609] -> w598
              frame #0 {
                n153 = local write "New Background Frame"(FALSE ("New Background")) -> ()
                n154 = local write "File Exists"(TRUE ("File Exists")) -> ()
              }
            }
          }
        }
      }
      event "New Background Movie": Value Change {
        n155 = event-data() -> ("NewVal"=w624:bool)  [unwired: 1 in]
        n156 = case shown="True" w624 {
          frame False {
          }
          frame True {
            n157 = flat-sequence {
              tunnel: [w644] -> w635
              tunnel: w634 -> [w643]
              tunnel: [w643] -> w633
              tunnel: [w642] -> w632
              tunnel: w629 -> [w641]
              tunnel: [w641] -> w628
              tunnel: w635 -> [w648]
              tunnel: w633 -> [w649]
              tunnel: w632 -> [w646]
              tunnel: [w648] -> w631
              tunnel: [w646] -> w630
              tunnel: w628 -> [w645]
              tunnel: [w645] -> w627
              tunnel: w631 -> [w655]
              tunnel: w630 -> [w654]
              tunnel: w627 -> [w652]
              tunnel: [w655] -> w626
              tunnel: [w654] -> w625
              tunnel: w626 -> [w656]
              tunnel: w625 -> [w657]
              frame #0 {
                n158 = local read "Manual Script Entry (0)"() -> (w644:string)
                n159 = local read "Script\n#"() -> (w642:i32)
                n160 = Wait (ms)(milliseconds to wait=u32 15) -> ()  [unwired: 1 out]
              }
              frame #1 {
                n161 = local write "Manual Script Entry (0)"(w649) -> ()
                n162 = local write "Script\n#"(0 ("Script\n#")) -> ()
              }
              frame #2 {
                n163 = Add(x=w652, y=500) -> (x+y=w650:i32)
                n164 = property on="SCRIPTING" class="Bool (strict)"("Val(Sgnl)"=TRUE ("Value (Signaling)")) -> ()  [unwired: 2 in, 2 out]
                n165 = Wait (ms)(milliseconds to wait=w650) -> ()  [unwired: 1 out]
              }
              frame #3 {
                n166 = local write "Manual Script Entry (0)"(w656) -> ()
                n167 = local write "Script\n#"(w657) -> ()
              }
              frame #4 {
                n168 = local write "New Background Movie"(FALSE ("New Background Movie")) -> ()
              }
            }
            n169 = local read "Cycle time\n(ms)"() -> (w638:i32)
            n170 = local read "# Frames"() -> (w637:i32)
            n171 = local read "MODE"() -> (w636:u16)
            n172 = local read "BIN"() -> (w639:u16)
            n173 = call "BGScriptGenerator.vi"("Cycle time\n(ms)"=w638, "# Frames"=w637, "BIN"=w639, "MODE"=w636) -> ("Duration (ms)"=w629:i32, "BG Script"=w634:string)  [unwired: 6 in]
          }
        }
      }
      event "Camera Set", "Mirror Set": Value Change {
        n174 = event-data() -> ("CtlRef"=w670:refnum<vi>)  [unwired: 1 in, 2 out]
        n175 = property class="DigNum (strict)"(reference=w670) -> ("Label.Text"=w669:string)  [unwired: 1 in, 2 out]
        n176 = case shown="\"Camera Set\"" w669 {
          tunnel: [2 ("Axis in") 1 ("Axis in")] -> w668
          tunnel: "Camera Set" -> [_ w683]
          tunnel: [w681 w683] -> w660
          tunnel: "Mirror Set" -> [w681 _]
          frame "Mirror Set", Default {
          }
          frame "Camera Set" {
          }
        }
        n177 = call <instrlib>:"Move absolute.vi"("error in"=w666, "New target position (units)"=w660, "Axis in"=w668, "VISA Handle in"=w667) -> ("error out"=w664:errorcluster, "VISA Handle out"=w665:refnum<visa-resource-name>, "TimeoutFlag"=w663:bool)  [unwired: 2 in, 1 out]
        n178 = local write "Translation Error"(w663) -> ()
      }
      event "Home": Value Change {
        n179 = event-data() -> ("NewVal"=w686:bool)  [unwired: 1 in]
        n180 = local read "Homing"() -> (w695:bool)
        n181 = Not(x=w695) -> (.not. x?=w696:bool)
        n182 = And(x=w686, y=w696) -> (x .and. y?=w697:bool)
        n183 = case shown="True" w697 {
          tunnel: w694 -> [w705 w718]
          tunnel: w693 -> [w704 w717]
          tunnel: [w704 w709] -> w687
          tunnel: [w705 w713] -> w688
          frame False {
          }
          frame True {
            n184 = call <instrlib>:"home.vi"("error in"=w717, "Axis in"=1, "VISA Handle in"=w718) -> ("error out"=w716:errorcluster, "VISA Handle out"=w714:refnum<visa-resource-name>, "TimeoutFlag"=w706:bool)  [unwired: 3 in, 1 out]
            n185 = flat-sequence {
              tunnel: w716 -> [w722]
              tunnel: [w722] -> w712
              frame #0 {
                n186 = Wait (ms)(milliseconds to wait=u32 50) -> ()  [unwired: 1 out]
              }
            }
            n187 = call <instrlib>:"home.vi"("error in"=w712, "Axis in"=2, "VISA Handle in"=w714) -> ("error out"=w710:errorcluster, "VISA Handle out"=w713:refnum<visa-resource-name>, "TimeoutFlag"=w707:bool)  [unwired: 3 in, 1 out]
            n188 = Or(x=w706, y=w707) -> (x .or. y?=w708:bool)
            n189 = local write "Translation Error"(w708) -> ()
            n190 = flat-sequence {
              tunnel: w710 -> [w720]
              tunnel: [w720] -> w709
              frame #0 {
                n191 = local write "Home"(FALSE ("Home")) -> ()
              }
            }
          }
        }
      }
      event "Initial Gate Delay (us)", "Second Gate Delay (us)", "Initial Gate Width (us)", "Second Gate Width (us)": Value Change {
        n192 = event-data() -> ()  [unwired: 1 in, 1 out]
        n193 = case shown="False" w724 {
          tunnel: w734 -> [w740 w744]
          tunnel: w733 -> [w739 w743]
          tunnel: [w739 w742] -> w726
          tunnel: [w740 w741] -> w725
          frame False {
          }
          frame True {
            w745 = 1000.0 ("Initial Gate Width (us)")
            n194 = Multiply(x="Initial Gate Delay (us)", y=w745) -> (x*y=w759:dbl)
            n195 = Multiply(x="Initial Gate Width (us)", y=w745) -> (x*y=w758:dbl)
            n196 = constructor class="Pulse"(error in=w743, "width"=w758, "delay"=w759) -> (reference out=w754:refnum<k24>, error out=w755:errorcluster)  [unwired: 2 in, 3 out]
            n197 = property class="CameraSettings"(error in=w755) -> (error out=w747:errorcluster, "GatingDifStartingGate"=w746:string)  [unwired: 1 in, 1 out]
            n198 = call <userlib>:"Adv_WriteLightFieldProperty.vi"("error in (no error)"=w747, "value"=w754, "setting"=w746, "LightField Automation in"=w744) -> ("error out"=w751:errorcluster, "LightField Automation out"=w749:refnum<class "LightField Automation.lvclass">)  [unwired: 6 in]
            n199 = Multiply(x="Second Gate Delay (us)", y=w745) -> (x*y=w763:dbl)
            n200 = Multiply(x="Second Gate Width (us)", y=w745) -> (x*y=w762:dbl)
            n201 = constructor class="Pulse"(error in=w751, "width"=w762, "delay"=w763) -> (reference out=w753:refnum<k24>, error out=w752:errorcluster)  [unwired: 2 in, 3 out]
            n202 = property class="CameraSettings"(error in=w752) -> (error out=w748:errorcluster, "GatingDifEndingGate"=w750:string)  [unwired: 1 in, 1 out]
            n203 = call <userlib>:"Adv_WriteLightFieldProperty.vi"("error in (no error)"=w748, "value"=w753, "setting"=w750, "LightField Automation in"=w749) -> ("error out"=w742:errorcluster, "LightField Automation out"=w741:refnum<class "LightField Automation.lvclass">)  [unwired: 6 in]
          }
        }
      }
    }
  }
  n204 = while {
    shift-right: [w864] -> w161
    shift-left: w160 -> [w863]
    shift-right: [w865] -> w162
    shift-left: w159 -> [w862]
    shift-right: [w859] -> w153
    shift-left: w157 -> [w861]
    shift-right: [w858] -> w152
    shift-left: w156 -> [w860]
    shift-right: [w857] -> w103
    shift-left: _ -> [w855]
    shift-right: [w856] -> w102
    shift-left: _ -> [w854]
    shift-right: [w851] -> w125
    shift-left: w134 -> [w853]
    shift-right: [w850] -> w127
    shift-left: w135 -> [w849]
    shift-right: [w847] -> w138
    shift-left: w147 -> [w848]
    shift-right: [w845] -> w139
    shift-left: w146 -> [w846]
    tunnel: w136 -> [w852]
    tunnel: [w821] -> w126
    shift-right: [w818] -> w107
    shift-left: w109 -> [w820]
    shift-right: [w817] -> w106
    shift-left: w108 -> [w819]
    shift-right: [w806] -> _
    shift-left: _ -> [w810]
    shift-right: [w805] -> w71
    shift-left: w69 -> [w802]
    shift-right: [w804] -> w72
    shift-left: w70 -> [w803]
    shift-right: [w796] -> w63
    shift-left: w67 -> [w799]
    shift-right: [w797] -> w62
    shift-left: w66 -> [w798]
    shift-right: [w790] -> _
    shift-left: _ -> [w792]
    shift-right: [w777] -> _
    shift-left: w48 -> [w779]
    shift-right: [w766] -> w12
    shift-left: w14 -> [w768]
    shift-right: [w767] -> w13
    shift-left: w15 -> [w769]
    stop <- w811 stop-if-true
    n205 = local read "DATA"() -> (w816:bool)
    n206 = Get Date/Time In Seconds() -> (seconds since 1Jan1904=w781:timestamp)
    n207 = call <instrlib>:"Collect Data.vi"("Location of FieldMax2Lib.dll in"=w819, "Meter ID in"=w820) -> ("Location of FieldMax2Lib.dll out"=w817:path, "Meter ID out"=w818:i32, "Measurement"=w814:sgl)  [unwired: 5 in, 1 out]
    n208 = Multiply(x="Data Interval (s)", y=u32 1000 ("millisecond multiple")) -> (x*y=w822:dbl)
    n209 = To Double Precision Float(number=w781) -> (double precision float=w777:dbl)
    n210 = Subtract(x=w777, y=w779) -> (x-y=w778:dbl)
    n211 = Multiply(x=w814, y=1000.0) -> (x*y=w813:dbl)
    "Power (mW)" <- w813
    n212 = Get Date/Time String(seconds (now)=w781, want seconds? (F)=TRUE) -> (time string=→"time string":string)  [unwired: 1 in, 1 out]
    n213 = call "Lakeshore218ReadTemp.vi"("error in"=w768, "VISA resource name"=w769) -> ("error out"=w766:errorcluster, "Thick Film R (Ohms)"=w770:string, "VISA resource name out"=w767:refnum<visa-resource-name>)  [unwired: 7 in]
    n214 = case shown="True" "RECORD" {
      tunnel: w855 -> [w919 _]
      tunnel: w854 -> [w920 _]
      tunnel: [w920 w925] -> w825
      tunnel: [w919 w924] -> w826
      frame False {
      }
      frame True {
        n215 = local read "SCRIPTING"() -> (w923:bool)
        n216 = local read "Script\n#"() -> (w922:i32)
        n217 = local write "RECORD"(FALSE ("RECORD")) -> ()
        n218 = call "DataHeader.vi"("Script #"=w922, "Scripting"=w923) -> ("error out"=w924:errorcluster, "Timestamp"=→"Timestamp":string, "refnum out"=w925:refnum<file>)  [unwired: 7 in]
      }
    }
    n219 = call "Lakeshore218Parse.vi"("Resistance String"=w770) -> ("Low Level (Ohms)"=w764:dbl, "High Level (Ohms)"=w765:dbl)  [unwired: 9 in]
    "High Level\n(Ohms)" <- w765
    "Low Level\n(Ohms)" <- w764
    n220 = call-poly <instrlib>:"Open.vi"("error in (no error)"=w862, "Device Identifier"="MB1.T1:TEMP", "Mercury Reference In"=w863) -> ("error out"=w838:errorcluster, "Mercury Reference Out"=w837:T5)  [unwired: 7 in]
    n221 = call-poly <instrlib>:"Signals (Read).vi"("error in"=w838, "Mercury Reference In"=w837) -> ("error out"=w835:errorcluster, "Temperature"=w789:dbl, "Mercury Reference Out"=w836:T5)  [unwired: 5 in, 2 out]
    "Cryostat (K)" <- w789
    n222 = call-poly <instrlib>:"Open.vi"("error in (no error)"=w835, "Device Identifier"="DB6.T1:TEMP", "Mercury Reference In"=w836) -> ("error out"=w833:errorcluster, "Mercury Reference Out"=w834:T5)  [unwired: 7 in]
    n223 = call "PressureControl - 3He.vi"("error in (no error)"=w848, "VISA resource name"=w846) -> ("error out"=w847:errorcluster, "3HePressure (Torr)"=w783:string, "VISA resource name out"=w845:refnum<visa-resource-name>)  [unwired: 7 in]
    n224 = call "PressureControl - 4He.vi"("error in (no error)"=w861, "VISA resource name"=w860) -> ("error out"=w859:errorcluster, "Pressure"=w828:dbl, "Pressure (Torr)"=w784:string, "VISA resource name out"=w858:refnum<visa-resource-name>)  [unwired: 6 in]
    n225 = call-poly <instrlib>:"Signals (Read).vi"("error in"=w833, "Mercury Reference In"=w834) -> ("error out"=w865:errorcluster, "Temperature"=w827:dbl, "Mercury Reference Out"=w864:T5)  [unwired: 5 in, 2 out]
    "Cell (K)" <- w827
    n226 = case shown="\"Fill Tanks\"" "Turbulence" {
      tunnel: w784 -> [w927 w930]
      tunnel: w783 -> [w928 w929]
      frame "Main Controls", Default {
        "Tank P2 (Torr)" <- w928
        "Tank P1 (Torr)" <- w927
      }
      frame "Fill Tanks" {
        n227 = event shown="[2] \"3He Pressure (Torr)\": Value Change" {
          selector: _ -> [_ _ _ _]
          dyn-events: _ -> [_ _ _ _]
          timeout: 500 ("Numeric") -> [_ _ _ _]
          tunnel: w929 -> [_ _ _ w936]
          tunnel: w930 -> [_ _ _ w938]
          event Timeout {
            n228 = event-data() -> ()  [unwired: 1 in, 3 out]
          }
          event "Desired Tank\nPressure (3He)": Value Change {
            n229 = event-data() -> ("NewVal"=w932:dbl)  [unwired: 1 in]
            n230 = call "3HePressureCalculator.vi"("Desired Tank\nPressure (3He)"=w932) -> ("V2 Pressure (3He)"=→"Desired V2\nPressure (3He)":dbl)  [unwired: 10 in]
          }
          event "3He Pressure (Torr)": Value Change {
            n231 = event-data() -> ("NewVal"=w934:string)  [unwired: 1 in]
            n232 = call "3HeActualPressure.vi"("3He Pressure (Torr)"=w934) -> ("Actual 3He\nTank Pressure"=→"Actual 3He\nTank Pressure":dbl)  [unwired: 10 in]
          }
          event "Log Pressure": Value Change {
            n233 = event-data() -> ("NewVal"=w937:bool)  [unwired: 1 in]
            n234 = call "SaveTankData.vi"("Log Pressure"=w937, "4He Pressure (Torr)"=w938, "3He Pressure (Torr)"=w936) -> ()  [unwired: 8 in]
          }
        }
        "3He Pressure (Torr)" <- w929
        "4He Pressure (Torr)" <- w930
      }
    }
    n235 = call-poly <vilib>:"DAQmx Read.vi"("task/channels in"=w803, "error in"=w802) -> ("task out"=w801:refnum<k21>, "data"=w806:dbl, "error out"=w800:errorcluster)  [unwired: 11 in]
    "Detected" <- w806
    n236 = call-poly <vilib>:"DAQmx Read.vi"("task/channels in"=w799, "error in"=w798) -> ("task out"=w795:refnum<k21>, "data"=w790:dbl, "error out"=w794:errorcluster)  [unwired: 11 in]
    "Incident" <- w790
    n237 = case shown="True" w816 {
      tunnel: w849 -> [w872 w908]
      tunnel: w853 -> [w874 w907]
      tunnel: w852 -> [w873 w906]
      tunnel: [w873 w902] -> w832
      tunnel: [w872 w901] -> w831
      tunnel: [w874 w900] -> w830
      tunnel: w827 -> [_ w882]
      tunnel: w789 -> [_ w887]
      tunnel: w826 -> [w870 w891]
      tunnel: w784 -> [_ w890]
      tunnel: w825 -> [w871 w892]
      tunnel: [w870 w879] -> w824
      tunnel: [w871 w880] -> w823
      tunnel: w822 -> [w869 w894]
      tunnel: [w869 w893] -> w812
      tunnel: w813 -> [_ w889]
      tunnel: w806 -> [_ w878]
      tunnel: w790 -> [_ w881]
      tunnel: "Top" -> [_ w886]
      tunnel: "Middle" -> [_ w888]
      tunnel: "Bottom" -> [_ w883]
      tunnel: w765 -> [_ w875]
      tunnel: w764 -> [_ w876]
      frame False {
      }
      frame True {
        n238 = Subtract(x=w894, y=350.0) -> (x-y=w893:dbl)
        n239 = call <instrlib>:"Measure.vi"("Function (Current)"=T7."Power", "error in (no error)"=w908, "Node In"=w906, "VISA resource name"=w907) -> ("error out"=w899:errorcluster, "Output"=w885:string, "Node Out"=w903:string, "VISA resource name out"=w904:refnum<visa-resource-name>)  [unwired: 3 in, 1 out]
        n240 = flat-sequence {
          tunnel: w899 -> [w909]
          tunnel: [w909] -> w898
          frame #0 {
            n241 = Wait (ms)(milliseconds to wait=u32 100) -> ()  [unwired: 1 out]
          }
        }
        n242 = local read "Liquid Level"() -> (w877:dbl)
        n243 = call <instrlib>:"Measure.vi"("Function (Current)"=T7."Power", "error in (no error)"=w898, "Channel (Channel A)"=Channel."Channel B", "Node In"=w903, "VISA resource name"=w904) -> ("error out"=w901:errorcluster, "Output"=w884:string, "Node Out"=w902:string, "VISA resource name out"=w900:refnum<visa-resource-name>)  [unwired: 2 in, 1 out]
        n244 = call "CompileData.vi"("refnum in"=w892, "Tank Pressure (Torr)"=w890, "Middle"=w888, "Laser Power (W)"=w889, "error in"=w891, "Cryostat Temp (K)"=w887, "Low Resistor"=w876, "High Resistor"=w875, "Ch. A (W)"=w885, "Top"=w886, "Bottom"=w883, "Cell Temp (K)"=w882, "Ch. B (W)"=w884, "Incident"=w881, "Liquid Level"=w877, "Detected"=w878) -> ("refnum out"=w880:refnum<file>, "error out"=w879:errorcluster)  [unwired: 2 in]
      }
    }
    n245 = case shown="True" "CLOSE" {
      tunnel: w824 -> [w911 w918]
      tunnel: w823 -> [w912 w917]
      tunnel: [w912 refnum<file> refnum ("refnum out")] -> w856
      tunnel: [w911 errorcluster {"status"=FALSE, "code"=0, "source"=""} ("error out")] -> w857
      frame False {
      }
      frame True {
        n246 = local write "CLOSE"(FALSE ("CLOSE")) -> ()
        n247 = Close File(refnum=w917, error in=w918) -> (error out=w913:errorcluster)  [unwired: 1 out]
        n248 = local write "Overall Error"(w913) -> ()
      }
    }
    n249 = Less?(x=w789, y=2.17) -> (x < y?=w786:bool)
    n250 = event shown="[0] Timeout" {
      selector: _ -> [_ _ _ _ _ _]
      dyn-events: _ -> [_ _ _ _ _ _]
      timeout: w812 -> [_ _ _ _ _ _]
      tunnel: w832 -> [w943 w957 w969 w981 w993 w1006]
      tunnel: w831 -> [w944 w958 w971 w983 w995 w1007]
      tunnel: w830 -> [w945 w956 w968 w980 w992 w1005]
      tunnel: [w945 w955 w970 w982 w994 w1005] -> w851
      tunnel: [w944 w951 w964 w978 w989 w1007] -> w850
      tunnel: [w943 w950 w963 w977 w988 w1006] -> w821
      tunnel: [w942 w949 w962 w976 w987 w1004] -> w805
      tunnel: [w941 w948 w961 w975 w986 w1003] -> w804
      tunnel: w801 -> [w941 w948 w961 w975 w986 w1002]
      tunnel: w800 -> [w942 w949 w962 w976 w987 w1001]
      tunnel: [w940 w947 w960 w974 w985 w999] -> w796
      tunnel: [w939 w946 w959 w973 w984 w998] -> w797
      tunnel: w795 -> [w940 w947 w960 w974 w985 w997]
      tunnel: w794 -> [w939 w946 w959 w973 w984 w996]
      event Timeout {
        n251 = event-data() -> ()  [unwired: 1 in, 3 out]
      }
      event "Top Coil (mA)": Value Change {
        n252 = event-data() -> ("NewVal"=w953:dbl)  [unwired: 1 in, 5 out]
        n253 = Divide(x=w953, y=1000.0) -> (x/y=w952:dbl)
        n254 = call <instrlib>:"Source Level.vi"("Level (0.000)"=w952, "error in (no error)"=w958, "Node In"=w957, "VISA resource name"=w956) -> ("error out"=w951:errorcluster, "Node Out"=w950:string, "VISA resource name out"=w955:refnum<visa-resource-name>)  [unwired: 4 in, 1 out]
      }
      event "Bottom Coil (mA)": Value Change {
        n255 = event-data() -> ("NewVal"=w966:dbl)  [unwired: 1 in, 5 out]
        n256 = Divide(x=w966, y=1000.0) -> (x/y=w965:dbl)
        n257 = call <instrlib>:"Source Level.vi"("Level (0.000)"=w965, "error in (no error)"=w971, "Channel (Channel A)"=Channel."Channel B", "Node In"=w969, "VISA resource name"=w968) -> ("error out"=w964:errorcluster, "Node Out"=w963:string, "VISA resource name out"=w970:refnum<visa-resource-name>)  [unwired: 3 in, 1 out]
      }
      event "Top Coil": Value Change {
        n258 = event-data() -> ("NewVal"=w979:bool)  [unwired: 1 in, 5 out]
        n259 = call <instrlib>:"Source Output Enable.vi"("Output (Off)"=w979, "error in (no error)"=w983, "Node In"=w981, "VISA resource name"=w980) -> ("error out"=w978:errorcluster, "Node Out"=w977:string, "VISA resource name out"=w982:refnum<visa-resource-name>)  [unwired: 4 in, 1 out]
      }
      event "Bottom Coil": Value Change {
        n260 = event-data() -> ("NewVal"=w990:bool)  [unwired: 1 in, 5 out]
        n261 = call <instrlib>:"Source Output Enable.vi"("Output (Off)"=w990, "error in (no error)"=w995, "Channel (Channel A)"=Channel."Channel B", "Node In"=w993, "VISA resource name"=w992) -> ("error out"=w989:errorcluster, "Node Out"=w988:string, "VISA resource name out"=w994:refnum<visa-resource-name>)  [unwired: 3 in, 1 out]
      }
      event "RESTART": Value Change {
        n262 = event-data() -> ("NewVal"=w1000:bool)  [unwired: 1 in, 5 out]
        n263 = case shown="True" w1000 {
          tunnel: w1002 -> [w1011 w1021]
          tunnel: w1001 -> [w1010 w1022]
          tunnel: [w1011 w1020] -> w1003
          tunnel: [w1010 w1019] -> w1004
          tunnel: [w1009 w1015] -> w999
          tunnel: [w1008 w1014] -> w998
          tunnel: w997 -> [w1009 w1013]
          tunnel: w996 -> [w1008 w1012]
          frame False {
          }
          frame True {
            n264 = call <vilib>:"DAQmx Stop Task.vi"("task/channels in"=w1021, "error in"=w1022) -> ("task out"=w1018:refnum<k21>, "error out"=w1023:errorcluster)  [unwired: 12 in]
            n265 = call <vilib>:"DAQmx Stop Task.vi"("task/channels in"=w1013, "error in"=w1012) -> ("task out"=w1016:refnum<k21>, "error out"=w1017:errorcluster)  [unwired: 12 in]
            n266 = local write "RESTART"(FALSE ("RESTART")) -> ()
            n267 = call <vilib>:"DAQmx Start Task.vi"("task/channels in"=w1018, "error in"=w1023) -> ("task out"=w1020:refnum<k21>, "error out"=w1019:errorcluster)  [unwired: 12 in]
            n268 = call <vilib>:"DAQmx Start Task.vi"("task/channels in"=w1016, "error in"=w1017) -> ("task out"=w1015:refnum<k21>, "error out"=w1014:errorcluster)  [unwired: 12 in]
          }
        }
      }
    }
    n269 = Subtract(x=w790, y=w792) -> (x-y=w791:dbl)
    n270 = Subtract(x=w806, y=w810) -> (x-y=w809:dbl)
    n271 = Less?(x=w828, y=24.5) -> (x < y?=w787:bool)
    n272 = And(x=w786, y=w787) -> (x .and. y?=w785:bool)
    n273 = Divide(x=w791, y=w778) -> (x/y=→"Rate (Hz)":dbl)
    n274 = Divide(x=w809, y=w778) -> (x/y=→"Rate (Hz)":dbl)
    n275 = case shown="True" w785 {
      tunnel: [FALSE ("RUN/STOP") TRUE ("RUN/STOP")] -> w774
      frame False {
      }
      frame True {
      }
    }
    n276 = property on="READY" class="Bool (strict)"() -> ("Value"=w776:bool)  [unwired: 2 in, 2 out]
    n277 = Equal?(x=w776, y=w774) -> (x = y?=w775:bool)
    n278 = case shown="False" w775 {
      tunnel: w774 -> [w866 _]
      frame False {
        n279 = property on="READY" class="Bool (strict)"("Val(Sgnl)"=w866) -> ()  [unwired: 2 in, 2 out]
      }
      frame True {
      }
    }
    n280 = local read "Kill Switch"() -> (w811:bool)
  }
  n281 = local write "3He Check"(TRUE ("3He Check")) -> ()
  n282 = call "LogHeader.vi"("Data folder"=path "C:/Data") -> ("error out"=w99:errorcluster, "refnum out"=w100:refnum<file>)  [unwired: 9 in]
  "Log" <- w100
  n283 = call "MFCInit.vi"() -> ("MFC error out"=w42:errorcluster, "MFC VISA out"=w41:refnum<visa-resource-name>)  [unwired: 10 in]
  n284 = local write "Error"(FALSE ("Error")) -> ()
  n285 = call "LevelProbeInit.vi"() -> ("error out"=w23:errorcluster, "VISA resource name out"=w22:refnum<visa-resource-name>)  [unwired: 9 in, 1 out]
  n286 = while {
    tunnel: [w1025] -> w35
    stop <- w1027 stop-if-true
    n287 = event shown="[1] \"FROM FILE\": Value Change" {
      selector: _ -> [_ _]
      dyn-events: _ -> [_ _]
      timeout: 500 -> [_ _]
      tunnel: [i32[] [] w1029] -> w1025
      event Timeout {
        n288 = event-data() -> ()  [unwired: 1 in, 3 out]
      }
      event "FROM FILE": Value Change {
        n289 = event-data() -> ("NewVal"=w1030:bool)  [unwired: 1 in]
        n290 = case shown="True" w1030 {
          tunnel: [i32[] [] w1032] -> w1029
          frame False {
          }
          frame True {
            n291 = call "ScriptReader.vi"("Script File"="Script File") -> ("Different Scripts"=w1034:i32, "Scripts"=w1035:i32[][])  [unwired: 9 in]
            n292 = for {
              N: w1034 -> [_]
              tunnel: w1035 -> [w1043] mode=indexing
              tunnel: [w1039] -> w1033 mode=indexing
              stop <- w1048 stop-if-true
              n293 = Index Array(array=w1043, index=0) -> (element=w1044:i32)
              n294 = Index Array(array=w1043, index=1) -> (element=w1042:i32)
              n295 = local write "Script\nEnd"(w1044) -> ()
              n296 = local write "Script\n#"(w1044) -> ()
              n297 = while {
                shift-right: [w1052] -> w1039
                shift-left: w1042 -> [w1050]
                stop <- w1057 stop-if-true
                n298 = flat-sequence {
                  tunnel: w1050 -> [w1060]
                  tunnel: [w1060] -> w1053
                  tunnel: w1053 -> [w1066]
                  tunnel: [w1063] -> w1052
                  frame #0 {
                    n299 = property on="SCRIPTING" class="Bool (strict)"("Val(Sgnl)"=TRUE ("Value (Signaling)")) -> ()  [unwired: 2 in, 2 out]
                    n300 = local write "Error"(FALSE ("Error")) -> ()
                  }
                  frame #1 {
                    n301 = while {
                      tunnel: [w1105] -> w1065
                      tunnel: w1066 -> [w1105]
                      tunnel: [w1104] -> w1064
                      tunnel: [w1099] -> w1062
                      stop <- w1101 stop-if-true
                      n302 = local read "FROM FILE"() -> (w1107:bool)
                      n303 = local read "SCRIPTING"() -> (w1100:bool)
                      n304 = local read "Kill Switch"() -> (w1106:bool)
                      n305 = local read "READY"() -> (w1109:bool)
                      n306 = Not(x=w1107) -> (.not. x?=w1108:bool)
                      n307 = Not(x=w1100) -> (.not. x?=w1099:bool)
                      n308 = Not(x=w1109) -> (.not. x?=w1104:bool)
                      n309 = Or(x=w1104, y=w1108) -> (x .or. y?=w1110:bool)
                      n310 = Or(x=w1110, y=w1106) -> (x .or. y?=w1102:bool)
                      n311 = Or(x=w1099, y=w1102) -> (x .or. y?=w1101:bool)
                      n312 = Wait (ms)(milliseconds to wait=u32 1000) -> ()  [unwired: 1 out]
                    }
                    n313 = case shown="True" w1064 {
                      tunnel: w1065 -> [w1069 w1077]
                      tunnel: [w1068 w1077] -> w1063
                      tunnel: w1062 -> [w1067 _]
                      frame False {
                        n314 = case shown="True" w1067 {
                          tunnel: w1069 -> [w1070 w1073]
                          tunnel: [w1070 w1072] -> w1068
                          frame False {
                          }
                          frame True {
                            n315 = Decrement(x=w1073) -> (x-1=w1072:i32)
                            n316 = Wait (ms)(milliseconds to wait=u32 13000) -> ()  [unwired: 1 out]
                          }
                        }
                      }
                      frame True {
                        n317 = local write "Error"(TRUE ("Error")) -> ()
                        n318 = while {
                          tunnel: [w1089] -> w1076
                          tunnel: [w1088] -> w1074
                          i -> [w1095]
                          stop <- w1096 stop-if-true
                          n319 = local read "Kill Switch"() -> (w1090:bool)
                          n320 = local read "FROM FILE"() -> (w1092:bool)
                          n321 = local read "READY"() -> (w1088:bool)
                          n322 = Equal?(x=w1095, y=60) -> (x = y?=w1089:bool)
                          n323 = Not(x=w1092) -> (.not. x?=w1091:bool)
                          n324 = Or(x=w1090, y=w1089) -> (x .or. y?=w1093:bool)
                          n325 = Or(x=w1091, y=w1093) -> (x .or. y?=w1097:bool)
                          n326 = Or(x=w1097, y=w1088) -> (x .or. y?=w1096:bool)
                          n327 = Wait (ms)(milliseconds to wait=u32 1000) -> ()  [unwired: 1 out]
                        }
                        n328 = case shown="False" w1076 {
                          selector: w1076 -> [_ w1080]
                          tunnel: w1074 -> [w1078 _]
                          frame False {
                            n329 = case shown="True" w1078 {
                              frame False {
                              }
                              frame True {
                                n330 = Wait (ms)(milliseconds to wait=u32 13000) -> ()  [unwired: 1 out]
                              }
                            }
                          }
                          frame True {
                            n331 = property on="COOLDOWN" class="Bool (strict)"("Val(Sgnl)"=w1080) -> ()  [unwired: 2 in, 2 out]
                            n332 = while {
                              stop <- w1086 stop-if-true
                              n333 = local read "Kill Switch"() -> (w1084:bool)
                              n334 = local read "READY"() -> (w1081:bool)
                              n335 = local read "FROM FILE"() -> (w1082:bool)
                              n336 = Not(x=w1082) -> (.not. x?=w1083:bool)
                              n337 = Or(x=w1081, y=w1084) -> (x .or. y?=w1085:bool)
                              n338 = Or(x=w1085, y=w1083) -> (x .or. y?=w1086:bool)
                              n339 = Wait (ms)(milliseconds to wait=u32 1000) -> ()  [unwired: 1 out]
                            }
                          }
                        }
                      }
                    }
                  }
                }
                n340 = local read "Kill Switch"() -> (w1058:bool)
                n341 = local read "FROM FILE"() -> (w1055:bool)
                n342 = Equal?(x=1, y=w1050) -> (x = y?=w1051:bool)
                n343 = Or(x=w1058, y=w1051) -> (x .or. y?=w1056:bool)
                n344 = Not(x=w1055) -> (.not. x?=w1054:bool)
                n345 = Or(x=w1056, y=w1054) -> (x .or. y?=w1057:bool)
              }
              n346 = local read "FROM FILE"() -> (w1040:bool)
              n347 = local read "Kill Switch"() -> (w1047:bool)
              n348 = Not(x=w1040) -> (.not. x?=w1041:bool)
              n349 = Or(x=w1041, y=w1047) -> (x .or. y?=w1048:bool)
            }
            n350 = flat-sequence {
              tunnel: w1033 -> [w1037]
              tunnel: [w1037] -> w1032
              frame #0 {
                n351 = property on="FROM FILE" class="Bool (strict)"("Val(Sgnl)"=FALSE ("Value (Signaling)")) -> ()  [unwired: 2 in, 2 out]
              }
            }
          }
        }
      }
    }
    n352 = local read "Kill Switch"() -> (w1027:bool)
  }
  n353 = while {
    shift-right: [w1121] -> w98
    shift-left: w100 -> [w1122]
    shift-right: [w1120] -> w97
    shift-left: w99 -> [w1123]
    shift-right: [w1114] -> w38
    shift-left: w41 -> [w1118]
    shift-right: [w1115] -> w39
    shift-left: w42 -> [w1119]
    shift-right: [w1116] -> _
    shift-left: 0.0 ("3He Pressure") -> [w1117]
    stop <- w1113 stop-if-true
    n354 = event shown="[3] Timeout" {
      selector: _ -> [_ _ _ _]
      dyn-events: _ -> [_ _ _ _]
      timeout: 500 -> [_ _ _ _]
      tunnel: w1123 -> [w1131 w1621 w1694 w1708]
      tunnel: w1122 -> [w1132 w1620 w1695 w1709]
      tunnel: [w1130 w1620 w1695 w1709] -> w1121
      tunnel: [w1129 w1621 w1694 w1708] -> w1120
      tunnel: w1119 -> [w1126 w1626 w1698 w1706]
      tunnel: w1118 -> [w1125 w1627 w1699 w1705]
      tunnel: w1117 -> [w1127 w1625 w1697 w1707]
      tunnel: [w1127 w1624 w1696 w1707] -> w1116
      tunnel: [w1126 w1623 w1698 w1706] -> w1115
      tunnel: [w1125 w1622 w1699 w1705] -> w1114
      event "SCRIPTING": Value Change {
        n355 = event-data() -> ()  [unwired: 1 in, 1 out]
        n356 = case shown="True" "SCRIPTING" {
          tunnel: w1132 -> [w1134 w1138]
          tunnel: w1131 -> [w1133 w1137]
          tunnel: [w1134 w1135] -> w1130
          tunnel: [w1133 w1136] -> w1129
          frame False {
          }
          frame True {
            n357 = local read "Script\n#"() -> (w1140:i32)
            n358 = Not Equal To 0?(x=w1140) -> (x != 0?=w1139:bool)
            n359 = case shown="True" w1139 {
              tunnel: w1138 -> [w1146 w1330]
              tunnel: w1137 -> [w1147 w1331]
              tunnel: [w1141 w1328] -> w1136
              tunnel: [w1142 w1329] -> w1135
              frame False {
                n360 = call "GetManualCommands.vi"("Manual Script Entry (0)"="Manual Script Entry (0)") -> ("Commands"=w1154:string[])  [unwired: 10 in]
                n361 = Array Size(array=w1154) -> (size(s)=w1150:i32)
                n362 = for {
                  tunnel: w1154 -> [w1186] mode=indexing
                  tunnel: [w1181] -> w1153
                  tunnel: [w1180] -> w1148
                  i -> [w1181]
                  stop <- w1183 stop-if-true
                  n363 = Match Pattern(string=w1186, regular expression="[a-z]+") -> (match substring=w1179:string, after substring=w1178:string)  [unwired: 1 in, 2 out]
                  n364 = call <vilib>:"Trim Whitespace.vi"("string"=w1178) -> ("trimmed string"=w1185:string)  [unwired: 1 in]
                  n365 = Concatenate Strings(w1179, w1178) -> (w1177:string)
                  n366 = case shown="\"data\"" w1179 {
                    tunnel: w1185 -> [_ w1199 w1218 w1233 w1240 w1258 w1276 w1305]
                    tunnel: [TRUE ("Top Coil") w1198 w1215 FALSE ("Top Coil") w1237 w1255 w1275 w1304] -> w1182
                    tunnel: w1181 -> [w1191 w1197 w1217 _ w1239 w1257 w1274 w1303]
                    tunnel: u32 0 ("Script Number") -> [w1190 w1196 w1216 _ w1238 w1256 w1273 w1302]
                    tunnel: [w1189 w1194 w1213 "" ("Error String") w1235 w1254 w1271 w1300] -> w1180
                    tunnel: w1177 -> [w1188 w1193 w1212 _ w1234 w1253 w1270 w1299]
                    frame "False", Default {
                      n367 = call "ErrorHandling.vi"("Bad Command"=w1188, "Line #"=w1191, "Script #"=w1190) -> ("Error String"=w1189:string)  [unwired: 8 in]
                    }
                    frame "data" {
                      n368 = case shown="\"False\", Default" w1199 {
                        tunnel: [FALSE ("DATA") TRUE ("DATA") FALSE ("DATA")] -> w1195
                        tunnel: [TRUE ("Top Coil") FALSE ("Top Coil") FALSE ("Top Coil")] -> w1198
                        tunnel: w1197 -> [w1202 _ _]
                        tunnel: w1196 -> [w1203 _ _]
                        tunnel: [w1201 "" ("Error String") "" ("Error String")] -> w1194
                        tunnel: w1193 -> [w1200 _ _]
                        frame "False", Default {
                          n369 = call "ErrorHandling.vi"("Bad Command"=w1200, "Line #"=w1202, "Script #"=w1203) -> ("Error String"=w1201:string)  [unwired: 8 in]
                        }
                        frame "on" {
                        }
                        frame "off" {
                        }
                      }
                      n370 = property on="DATA" class="Bool (strict)"("Val(Sgnl)"=w1195) -> ()  [unwired: 2 in, 2 out]
                    }
                    frame "pulse" {
                      n371 = case shown="\"False\", Default" w1218 {
                        tunnel: [FALSE ("Top Coil") TRUE ("Top Coil") w1229] -> w1214
                        tunnel: [TRUE FALSE w1229] -> w1215
                        tunnel: w1217 -> [w1222 _ _]
                        tunnel: w1216 -> [w1221 _ _]
                        tunnel: [w1220 "" ""] -> w1213
                        tunnel: w1212 -> [w1219 _ _]
                        frame "False", Default {
                          n372 = call "ErrorHandling.vi"("Bad Command"=w1219, "Line #"=w1222, "Script #"=w1221) -> ("Error String"=w1220:string)  [unwired: 8 in]
                        }
                        frame "on" {
                        }
                        frame "off" {
                          w1229 = FALSE ("Top Coil")
                        }
                      }
                      n373 = property on="RUN/STOP" class="Bool (strict)"("Val(Sgnl)"=w1214) -> ()  [unwired: 2 in, 2 out]
                    }
                    frame "wait" {
                      n374 = Decimal String To Number(string=w1233) -> (number=w1232:i32)  [unwired: 2 in, 1 out]
                      n375 = Wait (ms)(milliseconds to wait=w1232) -> ()  [unwired: 1 out]
                    }
                    frame "neutron" {
                      n376 = case shown="\"False\", Default" w1240 {
                        tunnel: w1239 -> [w1246 _ _]
                        tunnel: w1238 -> [w1245 _ _]
                        tunnel: [TRUE ("Top Coil") FALSE ("Top Coil") w1251] -> w1237
                        tunnel: [FALSE ("Neutron Shutter") TRUE ("Neutron Shutter") w1251] -> w1236
                        tunnel: [w1242 "" ("Error String") "" ("Error String")] -> w1235
                        tunnel: w1234 -> [w1241 _ _]
                        frame "False", Default {
                          n377 = call "ErrorHandling.vi"("Bad Command"=w1241, "Line #"=w1246, "Script #"=w1245) -> ("Error String"=w1242:string)  [unwired: 8 in]
                        }
                        frame "on" {
                        }
                        frame "off" {
                          w1251 = FALSE ("Neutron Shutter")
                        }
                      }
                      n378 = property on="Neutron Shutter" class="Bool (strict)"("Val(Sgnl)"=w1236) -> ()  [unwired: 2 in, 2 out]
                    }
                    frame "shutter" {
                      n379 = case shown="\"False\", Default" w1258 {
                        tunnel: w1257 -> [w1264 _ _]
                        tunnel: w1256 -> [w1263 _ _]
                        tunnel: [TRUE ("Top Coil") FALSE ("Top Coil") w1269] -> w1255
                        tunnel: [FALSE ("Neutron Shutter") TRUE ("Neutron Shutter") w1269] -> w1252
                        tunnel: [w1260 "" ("Error String") "" ("Error String")] -> w1254
                        tunnel: w1253 -> [w1259 _ _]
                        frame "False", Default {
                          n380 = call "ErrorHandling.vi"("Bad Command"=w1259, "Line #"=w1264, "Script #"=w1263) -> ("Error String"=w1260:string)  [unwired: 8 in]
                        }
                        frame "on" {
                        }
                        frame "off" {
                          w1269 = FALSE ("Neutron Shutter")
                        }
                      }
                      n381 = property on="Enable" class="Bool (strict)"("Val(Sgnl)"=w1252) -> ()  [unwired: 2 in, 2 out]
                    }
                    frame "coila" {
                      n382 = case shown="\"False\", Default" w1276 {
                        selector: w1276 -> [w1283 _]
                        tunnel: [w1285 w1298] -> w1272
                        tunnel: [w1284 w1298] -> w1275
                        tunnel: w1274 -> [w1280 _]
                        tunnel: w1273 -> [w1279 _]
                        tunnel: [w1278 "" ("Error String")] -> w1271
                        tunnel: w1270 -> [w1277 _]
                        frame "False", Default {
                          n383 = Match Pattern(string=w1283, regular expression="[^0-9.]") -> (offset past match=w1281:i32)  [unwired: 1 in, 3 out]
                          n384 = case shown="0, Default" w1281 {
                            tunnel: [FALSE ("Top Coil") TRUE ("Top Coil")] -> w1285
                            tunnel: [TRUE FALSE] -> w1284
                            tunnel: w1283 -> [_ w1294]
                            tunnel: w1280 -> [w1289 _]
                            tunnel: w1279 -> [w1288 _]
                            tunnel: [w1287 ""] -> w1278
                            tunnel: w1277 -> [w1286 _]
                            frame 0, Default {
                              n385 = call "ErrorHandling.vi"("Bad Command"=w1286, "Line #"=w1289, "Script #"=w1288) -> ("Error String"=w1287:string)  [unwired: 8 in]
                            }
                            frame -1 {
                              n386 = Fract/Exp String To Number(string=w1294) -> (number=w1293:dbl)  [unwired: 3 in, 1 out]
                              n387 = property on="Top Coil (mA)" class="DigNum (strict)"("Val(Sgnl)"=w1293) -> ()  [unwired: 2 in, 2 out]
                            }
                          }
                        }
                        frame "off" {
                          w1298 = FALSE ("Top Coil")
                        }
                      }
                      n388 = property on="Top Coil" class="Bool (strict)"("Val(Sgnl)"=w1272) -> ()  [unwired: 2 in, 2 out]
                    }
                    frame "coilb" {
                      n389 = case shown="\"False\", Default" w1305 {
                        selector: w1305 -> [w1312 _]
                        tunnel: [w1311 w1327] -> w1301
                        tunnel: [w1310 w1327] -> w1304
                        tunnel: w1303 -> [w1309 _]
                        tunnel: w1302 -> [w1308 _]
                        tunnel: [w1307 ""] -> w1300
                        tunnel: w1299 -> [w1306 _]
                        frame "False", Default {
                          n390 = Match Pattern(string=w1312, regular expression="[^0-9.]") -> (offset past match=w1313:i32)  [unwired: 1 in, 3 out]
                          n391 = case shown="0, Default" w1313 {
                            tunnel: w1312 -> [_ w1325]
                            tunnel: [FALSE TRUE] -> w1311
                            tunnel: [TRUE FALSE] -> w1310
                            tunnel: w1309 -> [w1318 _]
                            tunnel: w1308 -> [w1317 _]
                            tunnel: [w1316 ""] -> w1307
                            tunnel: w1306 -> [w1315 _]
                            frame 0, Default {
                              n392 = call "ErrorHandling.vi"("Bad Command"=w1315, "Line #"=w1318, "Script #"=w1317) -> ("Error String"=w1316:string)  [unwired: 8 in]
                            }
                            frame -1 {
                              n393 = Fract/Exp String To Number(string=w1325) -> (number=w1322:dbl)  [unwired: 3 in, 1 out]
                              n394 = property on="Bottom Coil (mA)" class="DigNum (strict)"("Val(Sgnl)"=w1322) -> ()  [unwired: 2 in, 2 out]
                            }
                          }
                        }
                        frame "off" {
                          w1327 = FALSE
                        }
                      }
                      n395 = property on="Bottom Coil" class="Bool (strict)"("Val(Sgnl)"=w1301) -> ()  [unwired: 2 in, 2 out]
                    }
                  }
                  n396 = local read "Kill Switch"() -> (w1176:bool)
                  n397 = Or(x=w1182, y=w1176) -> (x .or. y?=w1183:bool)
                }
                n398 = Decrement(x=w1150) -> (x-1=w1152:i32)
                n399 = Equal?(x=w1153, y=w1152) -> (x = y?=w1151:bool)
                n400 = case shown="False" w1151 {
                  tunnel: [w1170 w1173] -> w1149
                  tunnel: w1148 -> [w1168 _]
                  tunnel: [w1166 w1172] -> w1144
                  frame False {
                    w1165 = FALSE ("status")
                    n401 = property on="Bottom Coil" class="Bool (strict)"("Val(Sgnl)"=w1165) -> ()  [unwired: 2 in, 2 out]
                    n402 = property on="Neutron Shutter" class="Bool (strict)"("Val(Sgnl)"=w1165) -> ()  [unwired: 2 in, 2 out]
                    n403 = property on="Top Coil" class="Bool (strict)"("Val(Sgnl)"=w1165) -> ()  [unwired: 2 in, 2 out]
                    n404 = property on="Enable" class="Bool (strict)"("Val(Sgnl)"=w1165) -> ()  [unwired: 2 in, 2 out]
                    n405 = property on="RUN/STOP" class="Bool (strict)"("Val(Sgnl)"=w1165) -> ()  [unwired: 2 in, 2 out]
                    n406 = property on="DATA" class="Bool (strict)"("Val(Sgnl)"=w1165) -> ()  [unwired: 2 in, 2 out]
                    n407 = Concatenate Strings("Manual test failed!" ("Description"), "\r\n", w1168) -> (w1166:string)
                    n408 = Bundle("status"=w1165, "code"=1017, w1166) -> (w1170:cluster{"status":bool, "code":i32, string})  [unwired: 1 in]
                  }
                  frame True {
                    w1172 = "Manual test successful!" ("Description")
                    n409 = Bundle("status"=FALSE, "code"=0, "Description"=w1172) -> (w1173:T2)  [unwired: 1 in]
                  }
                }
                n410 = flat-sequence {
                  tunnel: w1149 -> [w1162]
                  tunnel: w1147 -> [w1158]
                  tunnel: w1146 -> [w1161]
                  tunnel: "Manual Script Entry (0)" -> [w1160]
                  tunnel: w1144 -> [w1159]
                  tunnel: [w1157] -> w1143
                  tunnel: [w1156] -> w1141
                  tunnel: w1143 -> [w1164]
                  tunnel: [w1164] -> w1142
                  frame #0 {
                    n411 = local write "Scripting Error"(w1162) -> ()
                    n412 = local read "Timestamp"() -> (w1155:string)
                    n413 = call "WriteResults_Manual.vi"("Timestamp"=w1155, "error in"=w1158, "Result"=w1159, "Commands"=w1160, "refnum in"=w1161) -> ("error out"=w1156:errorcluster, "refnum out"=w1157:refnum<file>)  [unwired: 5 in]
                  }
                  frame #1 {
                    n414 = property on="SCRIPTING" class="Bool (strict)"("Val(Sgnl)"=FALSE ("Value (Signaling)")) -> ()  [unwired: 2 in, 2 out]
                  }
                }
              }
              frame True {
                n415 = while {
                  tunnel: w1331 -> [w1337]
                  tunnel: w1330 -> [w1336]
                  tunnel: [w1335] -> w1329
                  tunnel: [w1333] -> w1328
                  stop <- w1332 stop-if-true
                  n416 = local read "Script\n#"() -> (w1339:i32)
                  n417 = call "GetCommands.vi"("Script Number"=w1339) -> ("Script Exists"=w1340:bool, "Commands"=w1341:string[], "Camera Settings"=w1342:dbl[], "Data Interval (s)"=w1338:dbl)  [unwired: 5 in]
                  n418 = case shown="True" w1340 {
                    tunnel: w1342 -> [_ w1380]
                    tunnel: w1341 -> [_ w1378]
                    tunnel: w1339 -> [w1359 w1376]
                    tunnel: w1338 -> [_ w1375]
                    tunnel: w1337 -> [w1353 w1373]
                    tunnel: w1336 -> [w1354 w1372]
                    tunnel: [w1352 w1371] -> w1335
                    tunnel: [w1351 w1370] -> w1334
                    frame False {
                      n419 = Number To Decimal String(number=w1359) -> (decimal integer string=w1358:string)  [unwired: 1 in]
                      n420 = Concatenate Strings("Script" ("string"), w1358, " does not exist." ("string")) -> (w1355:string)
                      n421 = Bundle("status"=FALSE, "code"=1017, w1355) -> (w1360:cluster{"status":bool, "code":i32, string})  [unwired: 1 in]
                      n422 = Get Date/Time In Seconds() -> (seconds since 1Jan1904=w1350:timestamp)
                      n423 = Format Date/Time String(time format string (%c)="%H:%M:%S", seconds (now)=w1350) -> (date/time string=w1348:string)  [unwired: 1 in]
                      n424 = local write "Scripting Error"(w1360) -> ()
                      n425 = call "WriteResults_Script.vi"("Timestamp"=w1348, "error in"=w1353, "Result"=w1355, "refnum in"=w1354) -> ("error out"=w1351:errorcluster, "refnum out"=w1352:refnum<file>)  [unwired: 6 in]
                      n426 = property on="SCRIPTING" class="Bool (strict)"("Val(Sgnl)"=FALSE ("Value (Signaling)")) -> ()  [unwired: 2 in, 2 out]
                    }
                    frame True {
                      n427 = flat-sequence {
                        tunnel: u32 100 ("milliseconds to wait") -> [w1389]
                        tunnel: w1380 -> [w1390]
                        tunnel: [w1390] -> w1369
                        tunnel: [w1389] -> w1368
                        tunnel: w1375 -> [w1388]
                        tunnel: w1369 -> [w1394]
                        tunnel: [w1394] -> w1387
                        tunnel: w1368 -> [w1393]
                        tunnel: [w1393] -> w1386
                        tunnel: w1387 -> [w1399]
                        tunnel: [w1399] -> w1385
                        tunnel: w1386 -> [w1398]
                        tunnel: [w1398] -> w1384
                        tunnel: w1385 -> [w1403]
                        tunnel: [w1403] -> w1367
                        tunnel: w1384 -> [w1402]
                        tunnel: [w1402] -> w1366
                        tunnel: w1367 -> [w1407]
                        tunnel: w1366 -> [w1408]
                        tunnel: [w1408] -> w1365
                        tunnel: [w1407] -> w1364
                        tunnel: [w1411] -> w1383
                        tunnel: w1365 -> [w1410]
                        tunnel: [w1410] -> w1382
                        tunnel: w1364 -> [w1411]
                        tunnel: w1383 -> [w1416]
                        tunnel: w1382 -> [w1415]
                        tunnel: w1378 -> [w1421]
                        tunnel: w1376 -> [w1420]
                        tunnel: [w1419] -> w1381
                        tunnel: [w1418] -> w1374
                        tunnel: w1377 -> [w1588]
                        tunnel: w1381 -> [w1589]
                        tunnel: w1376 -> [w1578]
                        tunnel: w1374 -> [w1585]
                        tunnel: w1373 -> [w1582]
                        tunnel: w1372 -> [w1583]
                        tunnel: [w1581] -> w1371
                        tunnel: [w1580] -> w1370
                        frame #0 {
                          n428 = property on="Data Interval (s)" class="DigNum (strict)"("Val(Sgnl)"=w1388) -> ()  [unwired: 2 in, 2 out]
                        }
                        frame #1 {
                          n429 = Index Array(array=w1394, index=0) -> (element=w1392:dbl)
                          n430 = To Unsigned Word Integer(number=w1392) -> (unsigned 16bit integer=w1391:u16)
                          n431 = local write "MODE"(w1391) -> ()
                        }
                        frame #2 {
                          n432 = Index Array(array=w1399, index=1) -> (element=w1397:dbl)
                          n433 = To Unsigned Word Integer(number=w1397) -> (unsigned 16bit integer=w1396:u16)
                          n434 = local write "BIN"(w1396) -> ()
                        }
                        frame #3 {
                          n435 = Index Array(array=w1403, index=2) -> (element=w1401:dbl)
                          n436 = local write "On CCD Acc."(w1401) -> ()
                        }
                        frame #4 {
                          n437 = Index Array(array=w1407, index=3) -> (element=w1405:dbl)
                          n438 = local write "Cycle time\n(ms)"(w1405) -> ()
                        }
                        frame #5 {
                          n439 = Index Array(array=w1411, index=4) -> (element=w1409:dbl)
                          n440 = property on="# Frames" class="DigNum (strict)"("Val(Sgnl)"=w1409) -> ()  [unwired: 2 in, 2 out]
                          n441 = Wait (ms)(milliseconds to wait=w1410) -> ()  [unwired: 1 out]
                        }
                        frame #6 {
                          n442 = Index Array(array=w1416, index=5) -> (element=w1414:dbl)
                          n443 = To Unsigned Word Integer(number=w1414) -> (unsigned 16bit integer=w1413:u16)
                          n444 = property on="Shutter Mode" class="Ring (strict)"("Val(Sgnl)"=w1413) -> ()  [unwired: 2 in, 2 out]
                          n445 = Wait (ms)(milliseconds to wait=w1415) -> ()  [unwired: 1 out]
                        }
                        frame #7 {
                          n446 = for {
                            tunnel: w1421 -> [w1433] mode=indexing
                            tunnel: w1420 -> [w1430]
                            tunnel: [w1427] -> w1419
                            tunnel: [w1426] -> w1418
                            i -> [w1427]
                            stop <- w1422 stop-if-true
                            n447 = Match Pattern(string=w1433, regular expression="[a-z]+") -> (match substring=w1425:string, after substring=w1424:string)  [unwired: 1 in, 2 out]
                            n448 = call <vilib>:"Trim Whitespace.vi"("string"=w1424) -> ("trimmed string"=w1431:string)  [unwired: 1 in]
                            n449 = Concatenate Strings(w1425, w1424) -> (w1423:string)
                            n450 = case shown="\"neutron\"" w1425 {
                              tunnel: w1431 -> [_ w1445 w1464 w1479 w1486 w1504 w1522 w1551]
                              tunnel: [TRUE ("Top Coil") w1444 w1461 FALSE ("Top Coil") w1483 w1501 w1521 w1550] -> w1429
                              tunnel: w1427 -> [w1437 w1443 w1463 _ w1485 w1503 w1520 w1549]
                              tunnel: w1430 -> [w1436 w1442 w1462 _ w1484 w1502 w1519 w1548]
                              tunnel: [w1434 w1440 w1459 "" ("Error String") w1481 w1500 w1517 w1546] -> w1426
                              tunnel: w1423 -> [w1435 w1439 w1458 _ w1480 w1499 w1516 w1545]
                              frame "False", Default {
                                n451 = call "ErrorHandling.vi"("Bad Command"=w1435, "Line #"=w1437, "Script #"=w1436) -> ("Error String"=w1434:string)  [unwired: 8 in]
                              }
                              frame "data" {
                                n452 = case shown="\"False\", Default" w1445 {
                                tunnel: [FALSE ("DATA") TRUE ("DATA") FALSE ("DATA")] -> w1441
                                tunnel: [TRUE ("Top Coil") FALSE ("Top Coil") FALSE ("Top Coil")] -> w1444
                                tunnel: w1443 -> [w1448 _ _]
                                tunnel: w1442 -> [w1449 _ _]
                                tunnel: [w1447 "" ""] -> w1440
                                tunnel: w1439 -> [w1446 _ _]
                                frame "False", Default {
                                n453 = call "ErrorHandling.vi"("Bad Command"=w1446, "Line #"=w1448, "Script #"=w1449) -> ("Error String"=w1447:string)  [unwired: 8 in]
                                }
                                frame "on" {
                                }
                                frame "off" {
                                }
                                }
                                n454 = property on="DATA" class="Bool (strict)"("Val(Sgnl)"=w1441) -> ()  [unwired: 2 in, 2 out]
                              }
                              frame "pulse" {
                                n455 = case shown="\"False\", Default" w1464 {
                                tunnel: [FALSE ("Top Coil") TRUE ("Top Coil") w1475] -> w1460
                                tunnel: [TRUE FALSE w1475] -> w1461
                                tunnel: w1463 -> [w1468 _ _]
                                tunnel: w1462 -> [w1467 _ _]
                                tunnel: [w1466 "" ("Error String") ""] -> w1459
                                tunnel: w1458 -> [w1465 _ _]
                                frame "False", Default {
                                n456 = call "ErrorHandling.vi"("Bad Command"=w1465, "Line #"=w1468, "Script #"=w1467) -> ("Error String"=w1466:string)  [unwired: 8 in]
                                }
                                frame "on" {
                                }
                                frame "off" {
                                w1475 = FALSE ("Top Coil")
                                }
                                }
                                n457 = property on="RUN/STOP" class="Bool (strict)"("Val(Sgnl)"=w1460) -> ()  [unwired: 2 in, 2 out]
                              }
                              frame "wait" {
                                n458 = Decimal String To Number(string=w1479) -> (number=w1478:i32)  [unwired: 2 in, 1 out]
                                n459 = Wait (ms)(milliseconds to wait=w1478) -> ()  [unwired: 1 out]
                              }
                              frame "neutron" {
                                n460 = case shown="\"False\", Default" w1486 {
                                tunnel: w1485 -> [w1492 _ _]
                                tunnel: w1484 -> [w1491 _ _]
                                tunnel: [TRUE ("Top Coil") FALSE ("Top Coil") w1497] -> w1483
                                tunnel: [FALSE ("Neutron Shutter") TRUE ("Neutron Shutter") w1497] -> w1482
                                tunnel: [w1488 "" ""] -> w1481
                                tunnel: w1480 -> [w1487 _ _]
                                frame "False", Default {
                                n461 = call "ErrorHandling.vi"("Bad Command"=w1487, "Line #"=w1492, "Script #"=w1491) -> ("Error String"=w1488:string)  [unwired: 8 in]
                                }
                                frame "on" {
                                }
                                frame "off" {
                                w1497 = FALSE ("Neutron Shutter")
                                }
                                }
                                n462 = property on="Neutron Shutter" class="Bool (strict)"("Val(Sgnl)"=w1482) -> ()  [unwired: 2 in, 2 out]
                              }
                              frame "shutter" {
                                n463 = case shown="\"off\"" w1504 {
                                tunnel: w1503 -> [w1510 _ _]
                                tunnel: w1502 -> [w1509 _ _]
                                tunnel: [TRUE ("Top Coil") FALSE ("Top Coil") w1515] -> w1501
                                tunnel: [FALSE ("Neutron Shutter") TRUE ("Neutron Shutter") w1515] -> w1498
                                tunnel: [w1506 "" ""] -> w1500
                                tunnel: w1499 -> [w1505 _ _]
                                frame "False", Default {
                                n464 = call "ErrorHandling.vi"("Bad Command"=w1505, "Line #"=w1510, "Script #"=w1509) -> ("Error String"=w1506:string)  [unwired: 8 in]
                                }
                                frame "on" {
                                }
                                frame "off" {
                                w1515 = FALSE ("Neutron Shutter")
                                }
                                }
                                n465 = property on="Enable" class="Bool (strict)"("Val(Sgnl)"=w1498) -> ()  [unwired: 2 in, 2 out]
                              }
                              frame "coila" {
                                n466 = case shown="\"False\", Default" w1522 {
                                selector: w1522 -> [w1529 _]
                                tunnel: [w1531 w1544] -> w1518
                                tunnel: [w1530 w1544] -> w1521
                                tunnel: w1520 -> [w1526 _]
                                tunnel: w1519 -> [w1525 _]
                                tunnel: [w1524 ""] -> w1517
                                tunnel: w1516 -> [w1523 _]
                                frame "False", Default {
                                n467 = Match Pattern(string=w1529, regular expression="[^0-9.]") -> (offset past match=w1527:i32)  [unwired: 1 in, 3 out]
                                n468 = case shown="-1" w1527 {
                                tunnel: [FALSE ("Top Coil") TRUE ("Top Coil")] -> w1531
                                tunnel: [TRUE FALSE] -> w1530
                                tunnel: w1529 -> [_ w1540]
                                tunnel: w1526 -> [w1535 _]
                                tunnel: w1525 -> [w1534 _]
                                tunnel: [w1533 ""] -> w1524
                                tunnel: w1523 -> [w1532 _]
                                frame 0, Default {
                                n469 = call "ErrorHandling.vi"("Bad Command"=w1532, "Line #"=w1535, "Script #"=w1534) -> ("Error String"=w1533:string)  [unwired: 8 in]
                                }
                                frame -1 {
                                n470 = Fract/Exp String To Number(string=w1540) -> (number=w1539:dbl)  [unwired: 3 in, 1 out]
                                n471 = property on="Top Coil (mA)" class="DigNum (strict)"("Val(Sgnl)"=w1539) -> ()  [unwired: 2 in, 2 out]
                                }
                                }
                                }
                                frame "off" {
                                w1544 = FALSE ("Top Coil")
                                }
                                }
                                n472 = property on="Top Coil" class="Bool (strict)"("Val(Sgnl)"=w1518) -> ()  [unwired: 2 in, 2 out]
                              }
                              frame "coilb" {
                                n473 = case shown="\"off\"" w1551 {
                                selector: w1551 -> [w1558 _]
                                tunnel: [w1557 w1573] -> w1547
                                tunnel: [w1556 w1573] -> w1550
                                tunnel: w1549 -> [w1555 _]
                                tunnel: w1548 -> [w1554 _]
                                tunnel: [w1553 "" ("Error String")] -> w1546
                                tunnel: w1545 -> [w1552 _]
                                frame "False", Default {
                                n474 = Match Pattern(string=w1558, regular expression="[^0-9.]") -> (offset past match=w1559:i32)  [unwired: 1 in, 3 out]
                                n475 = case shown="-1" w1559 {
                                tunnel: w1558 -> [_ w1571]
                                tunnel: [FALSE TRUE] -> w1557
                                tunnel: [TRUE FALSE] -> w1556
                                tunnel: w1555 -> [w1564 _]
                                tunnel: w1554 -> [w1563 _]
                                tunnel: [w1562 ""] -> w1553
                                tunnel: w1552 -> [w1561 _]
                                frame 0, Default {
                                n476 = call "ErrorHandling.vi"("Bad Command"=w1561, "Line #"=w1564, "Script #"=w1563) -> ("Error String"=w1562:string)  [unwired: 8 in]
                                }
                                frame -1 {
                                n477 = Fract/Exp String To Number(string=w1571) -> (number=w1568:dbl)  [unwired: 3 in, 1 out]
                                n478 = property on="Bottom Coil (mA)" class="DigNum (strict)"("Val(Sgnl)"=w1568) -> ()  [unwired: 2 in, 2 out]
                                }
                                }
                                }
                                frame "off" {
                                w1573 = FALSE
                                }
                                }
                                n479 = property on="Bottom Coil" class="Bool (strict)"("Val(Sgnl)"=w1547) -> ()  [unwired: 2 in, 2 out]
                              }
                            }
                            n480 = local read "Kill Switch"() -> (w1428:bool)
                            n481 = Or(x=w1429, y=w1428) -> (x .or. y?=w1422:bool)
                          }
                        }
                        frame #8 {
                          n482 = Decrement(x=w1588) -> (x-1=w1587:i32)
                          n483 = Equal?(x=w1589, y=w1587) -> (x = y?=w1577:bool)
                          n484 = local read "Error"() -> (w1574:bool)
                          n485 = Not(x=w1574) -> (.not. x?=w1575:bool)
                          n486 = And(x=w1577, y=w1575) -> (x .and. y?=w1576:bool)
                          n487 = case shown="False" w1576 {
                            tunnel: w1578 -> [w1601 w1608]
                            tunnel: [w1600 w1615] -> w1586
                            tunnel: w1585 -> [w1591 _]
                            tunnel: [w1595 w1609] -> w1584
                            tunnel: w1574 -> [_ _]
                            frame False {
                              w1594 = FALSE ("Value (Signaling)")
                              n488 = Equal?(x="", y=w1591) -> (x = y?=w1592:bool)
                              n489 = case shown="True" w1592 {
                                tunnel: w1591 -> [w1604 _]
                                tunnel: [w1604 "Temperature Warning!"] -> w1590
                                frame False {
                                }
                                frame True {
                                }
                              }
                              n490 = property on="Top Coil" class="Bool (strict)"("Val(Sgnl)"=w1594) -> ()  [unwired: 2 in, 2 out]
                              n491 = property on="Bottom Coil" class="Bool (strict)"("Val(Sgnl)"=w1594) -> ()  [unwired: 2 in, 2 out]
                              n492 = property on="SCRIPTING" class="Bool (strict)"("Val(Sgnl)"=w1594) -> ()  [unwired: 2 in, 2 out]
                              n493 = Number To Decimal String(number=w1601) -> (decimal integer string=w1598:string)  [unwired: 1 in]
                              n494 = property on="Neutron Shutter" class="Bool (strict)"("Val(Sgnl)"=w1594) -> ()  [unwired: 2 in, 2 out]
                              n495 = property on="DATA" class="Bool (strict)"("Val(Sgnl)"=w1594) -> ()  [unwired: 2 in, 2 out]
                              n496 = property on="RUN/STOP" class="Bool (strict)"("Val(Sgnl)"=w1594) -> ()  [unwired: 2 in, 2 out]
                              n497 = Concatenate Strings("Script" ("string"), w1598, " failed!" ("string"), "\r\n", w1590) -> (w1595:string)
                              n498 = property on="Enable" class="Bool (strict)"("Val(Sgnl)"=w1594) -> ()  [unwired: 2 in, 2 out]
                              n499 = Bundle(FALSE, 1017, w1595) -> (w1600:errorcluster)  [unwired: 1 in]
                            }
                            frame True {
                              n500 = Number To Decimal String(number=w1608) -> (decimal integer string=w1611:string)  [unwired: 1 in]
                              n501 = Less?(x=w1608, y="Script\nEnd") -> (x < y?=w1606:bool)
                              n502 = case shown="False" w1606 {
                                tunnel: w1608 -> [_ w1618]
                                frame False {
                                n503 = property on="SCRIPTING" class="Bool (strict)"("Val(Sgnl)"=FALSE ("Value (Signaling)")) -> ()  [unwired: 2 in, 2 out]
                                }
                                frame True {
                                n504 = Increment(x=w1618) -> (x+1=w1619:i32)
                                n505 = property on="Script\n#" class="DigNum (strict)"("Val(Sgnl)"=w1619) -> ()  [unwired: 2 in, 2 out]
                                n506 = Wait (ms)(milliseconds to wait=u32 5000) -> ()  [unwired: 1 out]
                                }
                              }
                              n507 = Concatenate Strings("Script" ("string"), w1611, " successful!" ("string")) -> (w1609:string)
                              n508 = Bundle(FALSE, 0, w1609) -> (w1615:errorcluster)  [unwired: 1 in]
                            }
                          }
                          "Scripting Error" <- w1586
                          n509 = local read "Timestamp"() -> (w1579:string)
                          n510 = call "WriteResults_Script.vi"("Timestamp"=w1579, "error in"=w1582, "Result"=w1584, "refnum in"=w1583) -> ("error out"=w1580:errorcluster, "refnum out"=w1581:refnum<file>)  [unwired: 6 in]
                        }
                      }
                      n511 = Array Size(array=w1378) -> (size(s)=w1377:i32)
                    }
                  }
                  n512 = flat-sequence {
                    tunnel: w1334 -> [w1345]
                    tunnel: [w1345] -> w1333
                    tunnel: [w1344] -> w1332
                    frame #0 {
                      n513 = local read "SCRIPTING"() -> (w1346:bool)
                      n514 = local read "Kill Switch"() -> (w1343:bool)
                      n515 = Not(x=w1346) -> (.not. x?=w1347:bool)
                      n516 = Or(x=w1347, y=w1343) -> (x .or. y?=w1344:bool)
                    }
                  }
                }
              }
            }
          }
        }
      }
      event "Fill": Value Change {
        n517 = event-data() -> ("NewVal"=w1628:bool)  [unwired: 1 in]
        n518 = case shown="True" w1628 {
          tunnel: w1626 -> [w1635 w1662]
          tunnel: w1627 -> [w1634 w1661]
          tunnel: [w1633 w1660] -> w1622
          tunnel: [w1632 w1659] -> w1623
          tunnel: w1625 -> [w1631 w1650]
          tunnel: [w1631 w1650] -> w1624
          frame False {
            n519 = flat-sequence {
              tunnel: w1635 -> [w1640]
              tunnel: w1634 -> [w1639]
              tunnel: [w1638] -> w1630
              tunnel: [w1637] -> w1629
              tunnel: [w1642] -> w1632
              tunnel: [w1643] -> w1633
              tunnel: w1630 -> [w1643]
              tunnel: w1629 -> [w1642]
              frame #0 {
                n520 = call "MFCSetpoint.vi"("MFC error in"=w1640, "MFC setpoint"=0.0, "MFC VISA in"=w1639) -> ("MFC error out"=w1637:errorcluster, "MFC VISA out"=w1638:refnum<visa-resource-name>)  [unwired: 7 in]
              }
              frame #1 {
                n521 = local write "3He Check"(TRUE ("3He Check")) -> ()
              }
            }
          }
          frame True {
            n522 = local read "Desired V2\nPressure (3He)"() -> (w1649:dbl)
            n523 = flat-sequence {
              tunnel: w1644 -> [w1664]
              tunnel: w1652 -> [w1665]
              tunnel: w1661 -> [w1666]
              tunnel: w1662 -> [w1667]
              tunnel: [w1667] -> w1648
              tunnel: [w1666] -> w1647
              tunnel: [w1665] -> w1646
              tunnel: [w1664] -> w1645
              tunnel: [w1671] -> w1658
              tunnel: [w1670] -> w1657
              tunnel: [w1668] -> w1654
              tunnel: w1648 -> [w1673]
              tunnel: w1647 -> [w1672]
              tunnel: w1646 -> [w1669]
              tunnel: w1645 -> [w1668]
              tunnel: w1658 -> [w1677]
              tunnel: w1657 -> [w1676]
              tunnel: [w1677] -> w1656
              tunnel: [w1676] -> w1655
              tunnel: w1654 -> [w1675]
              tunnel: w1651 -> [w1674]
              tunnel: [w1692] -> w1659
              tunnel: [w1693] -> w1660
              tunnel: w1656 -> [w1693]
              tunnel: w1655 -> [w1692]
              frame #0 {
                n524 = local write "3He Check"(FALSE ("3He Check")) -> ()
              }
              frame #1 {
                n525 = call "MFCSetpoint.vi"("MFC error in"=w1673, "MFC setpoint"=w1669, "MFC VISA in"=w1672) -> ("MFC error out"=w1670:errorcluster, "MFC VISA out"=w1671:refnum<visa-resource-name>)  [unwired: 7 in]
              }
              frame #2 {
                n526 = while {
                  tunnel: w1675 -> [w1690]
                  tunnel: w1674 -> [w1683]
                  i -> [w1686]
                  stop <- w1680 stop-if-true
                  n527 = local read "3He Pressure (Torr)"() -> (w1682:string)
                  n528 = Fract/Exp String To Number(string=w1682) -> (number=w1681:dbl)  [unwired: 3 in, 1 out]
                  n529 = Greater?(x=w1681, y=w1690) -> (0:w1689:bool)
                  n530 = Multiply(x=w1686, y=0.01) -> (x*y=w1685:dbl)
                  n531 = local read "Kill Switch"() -> (w1678:bool)
                  n532 = Greater?(x=w1685, y=w1683) -> (0:w1687:bool)
                  n533 = Or(x=w1687, y=w1689) -> (x .or. y?=w1679:bool)
                  n534 = Or(x=w1678, y=w1679) -> (x .or. y?=w1680:bool)
                  n535 = Wait (ms)(milliseconds to wait=u32 10) -> ()  [unwired: 1 out]
                }
              }
              frame #3 {
                n536 = property on="Fill" class="Bool (strict)"("Val(Sgnl)"=FALSE ("Value (Signaling)")) -> ()  [unwired: 2 in, 2 out]
              }
            }
            n537 = Add(x=w1650, y=w1649) -> (x+y=w1644:dbl)
            n538 = local read "Fill Time (s)"() -> (w1653:u32)
            n539 = call "MFCSettingCalc.vi"("Fill Time (s)"=w1653, "SetPoint"=w1649) -> ("Time (s)"=w1651:dbl, "MFC Setting"=w1652:dbl)  [unwired: 8 in]
          }
        }
      }
      event "Tare": Value Change {
        n540 = event-data() -> ("NewVal"=w1700:bool)  [unwired: 1 in]
        n541 = case shown="False" w1700 {
          tunnel: w1697 -> [w1701 _]
          tunnel: [w1701 w1702] -> w1696
          frame False {
          }
          frame True {
            n542 = local read "3He Pressure (Torr)"() -> (w1703:string)
            n543 = Fract/Exp String To Number(string=w1703) -> (number=w1702:dbl)  [unwired: 3 in, 1 out]
            n544 = local write "Tare"(FALSE ("Tare")) -> ()
          }
        }
      }
      event Timeout {
        n545 = event-data() -> ()  [unwired: 1 in, 3 out]
      }
    }
    n546 = local read "Kill Switch"() -> (w1111:bool)
    n547 = And(x=w1111, y="3He Check") -> (x .and. y?=w1113:bool)
  }
  n548 = while {
    shift-right: [w1710] -> w21
    shift-left: w22 -> [w1713]
    shift-right: [w1711] -> w20
    shift-left: w23 -> [w1712]
    stop <- w1715 stop-if-true
    n549 = event shown="[1] \"COOLDOWN\": Value Change" {
      selector: _ -> [_ _ _]
      dyn-events: _ -> [_ _ _]
      timeout: 500 -> [_ _ _]
      tunnel: [w1717 w1729 w1840] -> w1710
      tunnel: [w1716 w1728 w1841] -> w1711
      tunnel: w1713 -> [w1720 w1726 w1838]
      tunnel: w1712 -> [w1719 w1727 w1839]
      event Timeout {
        n550 = event-data() -> ()  [unwired: 1 in, 3 out]
        n551 = call "LevelProbeRead.vi"("error in"=w1719, "VISA resource name"=w1720) -> ("error out"=w1716:errorcluster, "% Full"=w1718:dbl, "VISA resource name out"=w1717:refnum<visa-resource-name>)  [unwired: 6 in, 1 out]
        "L-He Level" <- w1718
        n552 = local write "Liquid Level"(w1718) -> ()
        n553 = case shown="True" "AUTOFILL" {
          tunnel: w1718 -> [_ w1723]
          frame False {
          }
          frame True {
            n554 = Less?(x=w1723, y="Low Level") -> (x < y?=w1724:bool)
            n555 = case shown="True" w1724 {
              selector: w1724 -> [_ w1725]
              frame False {
              }
              frame True {
                n556 = property on="REFILL" class="Bool (strict)"("Val(Sgnl)"=w1725) -> ()  [unwired: 2 in, 2 out]
              }
            }
          }
        }
      }
      event "COOLDOWN": Value Change {
        n557 = event-data() -> ("NewVal"=w1730:bool)  [unwired: 1 in, 5 out]
        n558 = case shown="True" w1730 {
          tunnel: w1726 -> [w1732 w1760]
          tunnel: w1727 -> [w1731 w1759]
          tunnel: [w1732 w1737] -> w1729
          tunnel: [w1731 w1735] -> w1728
          frame False {
          }
          frame True {
            n559 = flat-sequence {
              tunnel: w1760 -> [w1761]
              tunnel: w1759 -> [w1762]
              tunnel: [w1762] -> w1758
              tunnel: [w1761] -> w1757
              tunnel: w1758 -> [w1764]
              tunnel: w1757 -> [w1765]
              tunnel: [w1765] -> w1755
              tunnel: [w1764] -> w1753
              tunnel: [w1773] -> w1756
              tunnel: w1755 -> [w1773]
              tunnel: [w1772] -> w1754
              tunnel: w1753 -> [w1772]
              tunnel: w1756 -> [w1777]
              tunnel: w1754 -> [w1776]
              tunnel: [w1777] -> w1752
              tunnel: [w1776] -> w1751
              tunnel: w1752 -> [w1781]
              tunnel: w1751 -> [w1780]
              tunnel: [w1781] -> w1750
              tunnel: [w1780] -> w1749
              tunnel: w1750 -> [w1793]
              tunnel: w1749 -> [w1794]
              tunnel: [w1791] -> w1748
              tunnel: [w1792] -> w1747
              tunnel: w1748 -> [w1798]
              tunnel: w1747 -> [w1797]
              tunnel: [w1796] -> w1746
              tunnel: [w1795] -> w1745
              tunnel: w1746 -> [w1814]
              tunnel: w1745 -> [w1815]
              tunnel: [w1813] -> w1744
              tunnel: [w1812] -> w1743
              tunnel: w1744 -> [w1816]
              tunnel: w1743 -> [w1817]
              tunnel: [w1817] -> w1742
              tunnel: [w1816] -> w1741
              tunnel: w1742 -> [w1820]
              tunnel: w1741 -> [w1819]
              tunnel: [w1820] -> w1740
              tunnel: [w1819] -> w1736
              tunnel: w1740 -> [w1828]
              tunnel: [w1828] -> w1738
              tunnel: w1736 -> [w1827]
              tunnel: [w1827] -> w1733
              tunnel: [w1832] -> w1739
              tunnel: w1738 -> [w1832]
              tunnel: [w1831] -> w1734
              tunnel: w1733 -> [w1831]
              tunnel: w1739 -> [w1836]
              tunnel: [w1836] -> w1737
              tunnel: [w1835] -> w1735
              tunnel: w1734 -> [w1835]
              frame #0 {
                n560 = property on="Percent Open" class="DigNum (strict)"("Val(Sgnl)"=100 ("Percent Open")) -> ()  [unwired: 2 in, 2 out]
              }
              frame #1 {
                n561 = while {
                  i -> [w1769]
                  stop <- w1766 stop-if-true
                  n562 = Greater Than 0?(x=w1769) -> (x > 0?=w1768:bool)
                  n563 = case shown="True" w1768 {
                    tunnel: [FALSE ("Motor free") w1771] -> w1766
                    frame False {
                    }
                    frame True {
                      n564 = local read "Motor free"() -> (w1771:bool)
                    }
                  }
                  n565 = Wait (ms)(milliseconds to wait=u32 50) -> ()  [unwired: 1 out]
                }
              }
              frame #2 {
                n566 = property on="Sample Space Pump" class="Bool (strict)"("Val(Sgnl)"=FALSE ("Sample Space Pump")) -> ()  [unwired: 2 in, 2 out]
                n567 = Wait (ms)(milliseconds to wait=u32 250) -> ()  [unwired: 1 out]
              }
              frame #3 {
                n568 = property on="Siphon Pump" class="Bool (strict)"("Val(Sgnl)"=TRUE ("Siphon Pump")) -> ()  [unwired: 2 in, 2 out]
                n569 = Wait (ms)(milliseconds to wait=u32 250) -> ()  [unwired: 1 out]
              }
              frame #4 {
                n570 = while {
                  stop <- w1785 stop-if-true
                  n571 = local read "Kill Switch"() -> (w1788:bool)
                  n572 = local read "COOLDOWN"() -> (w1783:bool)
                  n573 = property on="Cryostat (K)" class="DigNum (strict)"() -> ("Value"=w1790:dbl)  [unwired: 2 in, 2 out]
                  n574 = Not(x=w1783) -> (.not. x?=w1782:bool)
                  n575 = Less?(x=w1790, y=3.8) -> (x < y?=w1787:bool)
                  n576 = Or(x=w1788, y=w1787) -> (x .or. y?=w1784:bool)
                  n577 = Or(x=w1784, y=w1782) -> (x .or. y?=w1785:bool)
                  n578 = Wait (ms)(milliseconds to wait=u32 1000) -> ()  [unwired: 1 out]
                }
              }
              frame #5 {
                n579 = call "LevelProbeContinuous.vi"("error in"=w1794, "VISA resource name"=w1793) -> ("error out"=w1792:errorcluster, "VISA resource name out"=w1791:refnum<visa-resource-name>)  [unwired: 7 in, 1 out]
              }
              frame #6 {
                n580 = while {
                  shift-right: [w1803] -> w1795
                  shift-left: w1798 -> [w1804]
                  shift-right: [w1802] -> w1796
                  shift-left: w1797 -> [w1805]
                  stop <- w1806 stop-if-true
                  n581 = call "LevelProbeRead.vi"("error in"=w1805, "VISA resource name"=w1804) -> ("error out"=w1802:errorcluster, "% Full"=w1801:dbl, "VISA resource name out"=w1803:refnum<visa-resource-name>)  [unwired: 6 in, 1 out]
                  "Liquid Level" <- w1801
                  n582 = local read "COOLDOWN"() -> (w1810:bool)
                  n583 = local read "Kill Switch"() -> (w1807:bool)
                  n584 = local write "L-He Level"(w1801) -> ()
                  n585 = Greater?(x=w1801, y="High Level") -> (0:w1800:bool)
                  n586 = Not(x=w1810) -> (.not. x?=w1809:bool)
                  n587 = Or(x=w1800, y=w1807) -> (x .or. y?=w1808:bool)
                  n588 = Or(x=w1808, y=w1809) -> (x .or. y?=w1806:bool)
                  n589 = Wait (ms)(milliseconds to wait=u32 1000) -> ()  [unwired: 1 out]
                }
              }
              frame #7 {
                n590 = call "LevelProbeHold.vi"("error in"=w1814, "VISA resource name"=w1815) -> ("error out"=w1813:errorcluster, "VISA resource name out"=w1812:refnum<visa-resource-name>)  [unwired: 7 in, 1 out]
              }
              frame #8 {
                n591 = property on="Percent Open" class="DigNum (strict)"("Val(Sgnl)"=0 ("Percent Open")) -> ()  [unwired: 2 in, 2 out]
              }
              frame #9 {
                n592 = while {
                  i -> [w1824]
                  stop <- w1821 stop-if-true
                  n593 = Greater Than 0?(x=w1824) -> (x > 0?=w1823:bool)
                  n594 = case shown="True" w1823 {
                    tunnel: [FALSE ("Motor free") w1826] -> w1821
                    frame False {
                    }
                    frame True {
                      n595 = local read "Motor free"() -> (w1826:bool)
                    }
                  }
                  n596 = Wait (ms)(milliseconds to wait=u32 50) -> ()  [unwired: 1 out]
                }
              }
              frame #10 {
                n597 = property on="Sample Space Pump" class="Bool (strict)"("Val(Sgnl)"=TRUE ("Sample Space Pump")) -> ()  [unwired: 2 in, 2 out]
                n598 = Wait (ms)(milliseconds to wait=u32 250) -> ()  [unwired: 1 out]
              }
              frame #11 {
                n599 = property on="Siphon Pump" class="Bool (strict)"("Val(Sgnl)"=FALSE ("Siphon Pump")) -> ()  [unwired: 2 in, 2 out]
                n600 = Wait (ms)(milliseconds to wait=u32 250) -> ()  [unwired: 1 out]
              }
              frame #12 {
                n601 = property on="COOLDOWN" class="Bool (strict)"("Val(Sgnl)"=FALSE ("COOLDOWN")) -> ()  [unwired: 2 in, 2 out]
              }
            }
          }
        }
      }
      event "REFILL": Value Change {
        n602 = event-data() -> ("NewVal"=w1842:bool)  [unwired: 1 in, 5 out]
        n603 = case shown="True" w1842 {
          tunnel: w1838 -> [w1843 w1869]
          tunnel: w1839 -> [w1844 w1864]
          tunnel: [w1844 w1849] -> w1841
          tunnel: [w1843 w1854] -> w1840
          frame False {
          }
          frame True {
            n604 = flat-sequence {
              tunnel: [w1872] -> w1870
              tunnel: w1869 -> [w1872]
              tunnel: [w1871] -> w1865
              tunnel: w1864 -> [w1871]
              tunnel: w1870 -> [w1875]
              tunnel: [w1875] -> w1867
              tunnel: w1865 -> [w1874]
              tunnel: [w1874] -> w1861
              tunnel: [w1883] -> w1868
              tunnel: w1867 -> [w1883]
              tunnel: [w1882] -> w1862
              tunnel: w1861 -> [w1882]
              tunnel: w1868 -> [w1887]
              tunnel: [w1887] -> w1866
              tunnel: [w1886] -> w1863
              tunnel: w1862 -> [w1886]
              tunnel: w1866 -> [w1892]
              tunnel: w1863 -> [w1893]
              tunnel: [w1891] -> w1860
              tunnel: [w1890] -> w1859
              tunnel: w1860 -> [w1897]
              tunnel: w1859 -> [w1896]
              tunnel: [w1895] -> w1858
              tunnel: [w1894] -> w1857
              tunnel: w1858 -> [w1914]
              tunnel: w1857 -> [w1913]
              tunnel: [w1911] -> w1856
              tunnel: [w1912] -> w1855
              tunnel: w1856 -> [w1916]
              tunnel: w1855 -> [w1915]
              tunnel: [w1916] -> w1850
              tunnel: [w1915] -> w1845
              tunnel: [w1919] -> w1851
              tunnel: w1850 -> [w1919]
              tunnel: [w1918] -> w1846
              tunnel: w1845 -> [w1918]
              tunnel: [w1927] -> w1852
              tunnel: w1851 -> [w1927]
              tunnel: [w1926] -> w1847
              tunnel: w1846 -> [w1926]
              tunnel: [w1931] -> w1853
              tunnel: w1852 -> [w1931]
              tunnel: [w1930] -> w1848
              tunnel: w1847 -> [w1930]
              tunnel: [w1935] -> w1854
              tunnel: w1853 -> [w1935]
              tunnel: [w1934] -> w1849
              tunnel: w1848 -> [w1934]
              frame #0 {
                n605 = property on="Percent Open" class="DigNum (strict)"("Val(Sgnl)"=100 ("Percent Open")) -> ()  [unwired: 2 in, 2 out]
              }
              frame #1 {
                n606 = while {
                  i -> [w1879]
                  stop <- w1876 stop-if-true
                  n607 = Greater Than 0?(x=w1879) -> (x > 0?=w1878:bool)
                  n608 = case shown="True" w1878 {
                    tunnel: [FALSE ("Motor free") w1881] -> w1876
                    frame False {
                    }
                    frame True {
                      n609 = local read "Motor free"() -> (w1881:bool)
                    }
                  }
                  n610 = Wait (ms)(milliseconds to wait=u32 50) -> ()  [unwired: 1 out]
                }
              }
              frame #2 {
                n611 = property on="Sample Space Pump" class="Bool (strict)"("Val(Sgnl)"=FALSE ("Sample Space Pump")) -> ()  [unwired: 2 in, 2 out]
                n612 = Wait (ms)(milliseconds to wait=u32 100) -> ()  [unwired: 1 out]
              }
              frame #3 {
                n613 = property on="Siphon Pump" class="Bool (strict)"("Val(Sgnl)"=TRUE ("Siphon Pump")) -> ()  [unwired: 2 in, 2 out]
                n614 = Wait (ms)(milliseconds to wait=u32 100) -> ()  [unwired: 1 out]
              }
              frame #4 {
                n615 = call "LevelProbeContinuous.vi"("error in"=w1893, "VISA resource name"=w1892) -> ("error out"=w1890:errorcluster, "VISA resource name out"=w1891:refnum<visa-resource-name>)  [unwired: 7 in, 1 out]
              }
              frame #5 {
                n616 = while {
                  shift-right: [w1902] -> w1895
                  shift-left: w1897 -> [w1903]
                  shift-right: [w1901] -> w1894
                  shift-left: w1896 -> [w1904]
                  stop <- w1905 stop-if-true
                  n617 = call "LevelProbeRead.vi"("error in"=w1904, "VISA resource name"=w1903) -> ("error out"=w1901:errorcluster, "% Full"=w1899:dbl, "VISA resource name out"=w1902:refnum<visa-resource-name>)  [unwired: 6 in, 1 out]
                  n618 = local read "High Level"() -> (w1898:dbl)
                  n619 = local write "L-He Level"(w1899) -> ()
                  n620 = local write "Liquid Level"(w1899) -> ()
                  n621 = local read "AUTOFILL"() -> (w1909:bool)
                  n622 = Greater?(x=w1899, y=w1898) -> (0:w1900:bool)
                  n623 = local read "Kill Switch"() -> (w1906:bool)
                  n624 = Wait (ms)(milliseconds to wait=u32 1000) -> ()  [unwired: 1 out]
                  n625 = Not(x=w1909) -> (.not. x?=w1908:bool)
                  n626 = Or(x=w1900, y=w1906) -> (x .or. y?=w1907:bool)
                  n627 = Or(x=w1907, y=w1908) -> (x .or. y?=w1905:bool)
                }
              }
              frame #6 {
                n628 = call "LevelProbeHold.vi"("error in"=w1913, "VISA resource name"=w1914) -> ("error out"=w1912:errorcluster, "VISA resource name out"=w1911:refnum<visa-resource-name>)  [unwired: 7 in, 1 out]
              }
              frame #7 {
                n629 = property on="Percent Open" class="DigNum (strict)"("Val(Sgnl)"=0 ("Percent Open")) -> ()  [unwired: 2 in, 2 out]
              }
              frame #8 {
                n630 = while {
                  i -> [w1923]
                  stop <- w1920 stop-if-true
                  n631 = Greater Than 0?(x=w1923) -> (x > 0?=w1922:bool)
                  n632 = case shown="True" w1922 {
                    tunnel: [FALSE ("Motor free") w1925] -> w1920
                    frame False {
                    }
                    frame True {
                      n633 = local read "Motor free"() -> (w1925:bool)
                    }
                  }
                  n634 = Wait (ms)(milliseconds to wait=u32 50) -> ()  [unwired: 1 out]
                }
              }
              frame #9 {
                n635 = property on="Sample Space Pump" class="Bool (strict)"("Val(Sgnl)"=TRUE ("Sample Space Pump")) -> ()  [unwired: 2 in, 2 out]
                n636 = Wait (ms)(milliseconds to wait=u32 100) -> ()  [unwired: 1 out]
              }
              frame #10 {
                n637 = property on="Siphon Pump" class="Bool (strict)"("Val(Sgnl)"=FALSE ("Siphon Pump")) -> ()  [unwired: 2 in, 2 out]
                n638 = Wait (ms)(milliseconds to wait=u32 100) -> ()  [unwired: 1 out]
              }
              frame #11 {
                n639 = property on="REFILL" class="Bool (strict)"("Val(Sgnl)"=FALSE ("COOLDOWN")) -> ()  [unwired: 2 in, 2 out]
              }
            }
          }
        }
      }
    }
    n640 = local read "Kill Switch"() -> (w1715:bool)
  }
  n641 = VISA Close(VISA resource name=w30, error in (no error)=w29) -> (error out=w28:errorcluster)
  n642 = VISA Close(VISA resource name=w13, error in (no error)=w12) -> (error out=w11:errorcluster)
  n643 = flat-sequence {
    tunnel: w55 -> [w1938]
    tunnel: [w1938] -> w54
    tunnel: [w1937] -> w53
    frame #0 {
      n644 = local read "LIGHTFIELD"() -> (w1937:bool)
    }
  }
  n645 = call "NeedleValveClose.vi"("error in (no error)"=w148, "VISA resource name"=w149) -> ("error out"=w78:errorcluster, "VISA resource name out"=w80:refnum<visa-resource-name>)  [unwired: 8 in]
  n646 = call "RelayControl.vi"("Neutron Shutter"=w101, "Error In"=w121, "Sample Space Pump"=w101, "Siphon Pump"=w101, "Relay In"=w119) -> ("Error Out"=w120:errorcluster, "Relay Out"=w118:refnum<visa-resource-name>)  [unwired: 5 in]
  n647 = flat-sequence {
    tunnel: [w1940] -> w50
    tunnel: w51 -> [w1940]
    tunnel: [w1939] -> w49
    frame #0 {
      n648 = local read "Enable"() -> (w1939:bool)
    }
  }
  n649 = flat-sequence {
    tunnel: [w1944] -> w114
    tunnel: [w1943] -> w115
    tunnel: w116 -> [w1942]
    tunnel: w117 -> [w1941]
    frame #0 {
      n650 = VISA Write(VISA resource name=w1942, write buffer=":PULSE0:STATE OFF\r\n" ("format string"), error in (no error)=w1941) -> (VISA resource name out=w1943:refnum<visa-resource-name>, error out=w1944:errorcluster)  [unwired: 1 out]
    }
  }
  n651 = VISA Close(VISA resource name=w118, error in (no error)=w120) -> (error out=w113:errorcluster)
  n652 = flat-sequence {
    tunnel: w78 -> [w1946]
    tunnel: [w1946] -> w81
    tunnel: [w1949] -> w79
    tunnel: w81 -> [w1949]
    frame #0 {
      n653 = Wait (ms)(milliseconds to wait=u32 3000) -> ()  [unwired: 1 out]
    }
    frame #1 {
      n654 = local write "Percent Open"(0 ("Percent Open")) -> ()
    }
  }
  n655 = case shown="True" w49 {
    tunnel: [w1951 w1955] -> w59
    tunnel: [w1950 w1954] -> w58
    tunnel: w57 -> [w1950 w1953]
    tunnel: w50 -> [w1951 w1952]
    frame False {
    }
    frame True {
      n656 = call "ToggleShutter.vi"("error in"=w1952, "VISA resource name"=w1953) -> ("error out"=w1955:errorcluster, "VISA resource name out"=w1954:refnum<visa-resource-name>)  [unwired: 8 in]
    }
  }
  n657 = flat-sequence {
    tunnel: w101 -> [w1957]
    tunnel: [w1958] -> w26
    tunnel: w113 -> [w1958]
    tunnel: w28 -> [w1956]
    tunnel: [w1956] -> w27
    frame #0 {
      n658 = local write "Siphon Pump"(w1957) -> ()
      n659 = local write "Sample Space Pump"(w1957) -> ()
      n660 = local write "Neutron Shutter"(w1957) -> ()
    }
  }
  n661 = Equal?(x=w53, y=TRUE) -> (x = y?=w60:bool)
  n662 = call <vilib>:"DAQmx Stop Task.vi"("task/channels in"=w72, "error in"=w71) -> ()  [unwired: 12 in, 2 out]
  n663 = call <vilib>:"DAQmx Stop Task.vi"("task/channels in"=w63, "error in"=w62) -> ()  [unwired: 12 in, 2 out]
  n664 = call <instrlib>:"Close.vi"("error in (no error)"=w162, "Mercury Reference"=w161) -> ("error out"=w129:errorcluster)  [unwired: 9 in]
  n665 = call <instrlib>:"Disconnect From Meter.vi"("Location of FieldMax2Lib.dll in"=w106, "Meter ID in"=w107) -> ()  [unwired: 7 in, 2 out]
  n666 = VISA Close(VISA resource name=w58, error in (no error)=w59) -> (error out=w56:errorcluster)
  n667 = call "KeithleyClose.vi"("Keithley Error In"=w127, "Node In"=w126, "KeithleyVISA In"=w125) -> ("Heater Error"=w124:errorcluster)  [unwired: 8 in]
  n668 = VISA Close(VISA resource name=w152, error in (no error)=w153) -> (error out=w10:errorcluster)
  n669 = call "3HeClose.vi"("error in (no error)"=w138, "VISA resource name"=w139) -> ("error out"=w6:errorcluster)  [unwired: 9 in]
  n670 = Not Equal?(x=refnum<file> refnum, y=w102) -> (x != y?=w104:bool)
  n671 = Merge Errors(w11, w10) -> (w5:errorcluster)
  n672 = Merge Errors(w26, w27) -> (w3:errorcluster)
  n673 = VISA Close(VISA resource name=w21, error in (no error)=w20) -> (error out=w19:errorcluster)
  n674 = case shown="True" w60 {
    tunnel: w61 -> [w1959 w1963]
    tunnel: w54 -> [_ w1962]
    tunnel: [w1959 w1960] -> w2
    frame False {
    }
    frame True {
      n675 = call <userlib>:"Adv_Deregister_for_Callback.vi"("error in (no error)"=w1963, "LightField Automation in"=w1962) -> ("error out"=w1964:errorcluster, "LightField Automation out"=w1965:refnum<class "LightField Automation.lvclass">)  [unwired: 8 in]
      n676 = call <userlib>:"LFA_Close.vi"("error in (no error)"=w1964, "LightField Automation in"=w1965) -> ("error out"=w1961:errorcluster)  [unwired: 8 in, 1 out]
      n677 = flat-sequence {
        tunnel: w1961 -> [w1967]
        tunnel: [w1967] -> w1960
        frame #0 {
          n678 = local write "LIGHTFIELD"(FALSE ("LIGHTFIELD")) -> ()
        }
      }
    }
  }
  n679 = VISA Close(VISA resource name=w115, error in (no error)=w114) -> (error out=w4:errorcluster)
  n680 = flat-sequence {
    tunnel: w124 -> [w1969]
    tunnel: [w1969] -> w8
    frame #0 {
      w1968 = FALSE ("Top Coil")
      n681 = local write "Top Coil"(w1968) -> ()
      n682 = local write "Bottom Coil"(w1968) -> ()
    }
  }
  n683 = VISA Close(VISA resource name=w80, error in (no error)=w79) -> (error out=w128:errorcluster)
  n684 = flat-sequence {
    tunnel: w56 -> [w1971]
    tunnel: [w1971] -> w1
    frame #0 {
      n685 = local write "Enable"(FALSE ("Enable")) -> ()
    }
  }
  n686 = case shown="True" w104 {
    tunnel: w103 -> [w1972 w1975]
    tunnel: w102 -> [_ w1974]
    tunnel: [w1972 w1973] -> w7
    frame False {
    }
    frame True {
      n687 = Close File(refnum=w1974, error in=w1975) -> (error out=w1973:errorcluster)  [unwired: 1 out]
    }
  }
  n688 = flat-sequence {
    tunnel: w129 -> [w1986]
    tunnel: w128 -> [w1987]
    tunnel: [w1991] -> w95
    tunnel: w96 -> [w1991]
    tunnel: w37 -> [w1981]
    tunnel: w35 -> [w1989]
    tunnel: [w1989] -> _
    tunnel: w19 -> [w1980]
    tunnel: [w1988] -> w9
    tunnel: w8 -> [w1985]
    tunnel: w7 -> [w1984]
    tunnel: w6 -> [w1983]
    tunnel: w5 -> [w1982]
    tunnel: w4 -> [w1979]
    tunnel: w3 -> [w1978]
    tunnel: w2 -> [w1977]
    tunnel: w1 -> [w1976]
    frame #0 {
      w1990 = FALSE ("Kill Switch")
      n689 = Merge Errors(w1986, w1987, w1985, w1984, w1983, w1982, w1981, w1980, w1979, w1978, w1977, w1976) -> (w1988:errorcluster)
      n690 = local write "Kill Switch"(w1990) -> ()
      n691 = local write "READY"(w1990) -> ()
      n692 = local write "LIGHTFIELD"(w1990) -> ()
    }
  }
  n693 = VISA Close(VISA resource name=w38, error in (no error)=w39) -> (error out=w37:errorcluster)
  n694 = Close File(refnum=w98, error in=w97) -> (error out=w96:errorcluster)  [unwired: 1 out]
  "Overall Error" <- w9
  "Log Error" <- w95
